vi "BRig_RT__Case_Exp__State_initTrial__LC_ENL__v18.vi"(6 "input_arrTrig":bool[](array[boolean]), 8 "input_dataTrial":u16[][](array[numeric]), 9 "input_dataExp":u16[](array[numeric]), 10 "input_dataLC":u16[](array[numeric]), 11 "input_dataCurrent":u16[](array[numeric])) -> (0 "output_dataTrial":u16[][](array[numeric]), 3 "output_dataCurrent":u16[](array[numeric]), 4 "output_arrTrig":bool[](array[boolean]))   [LabVIEW 2014]
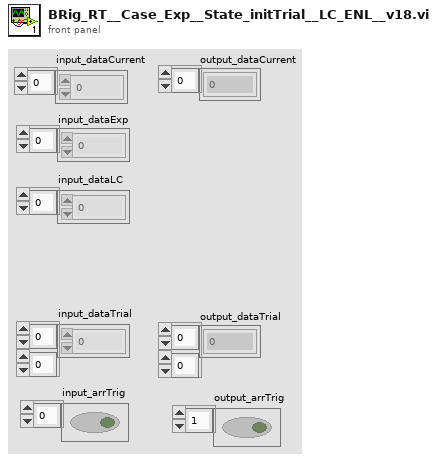
[diagram p1: front panel]
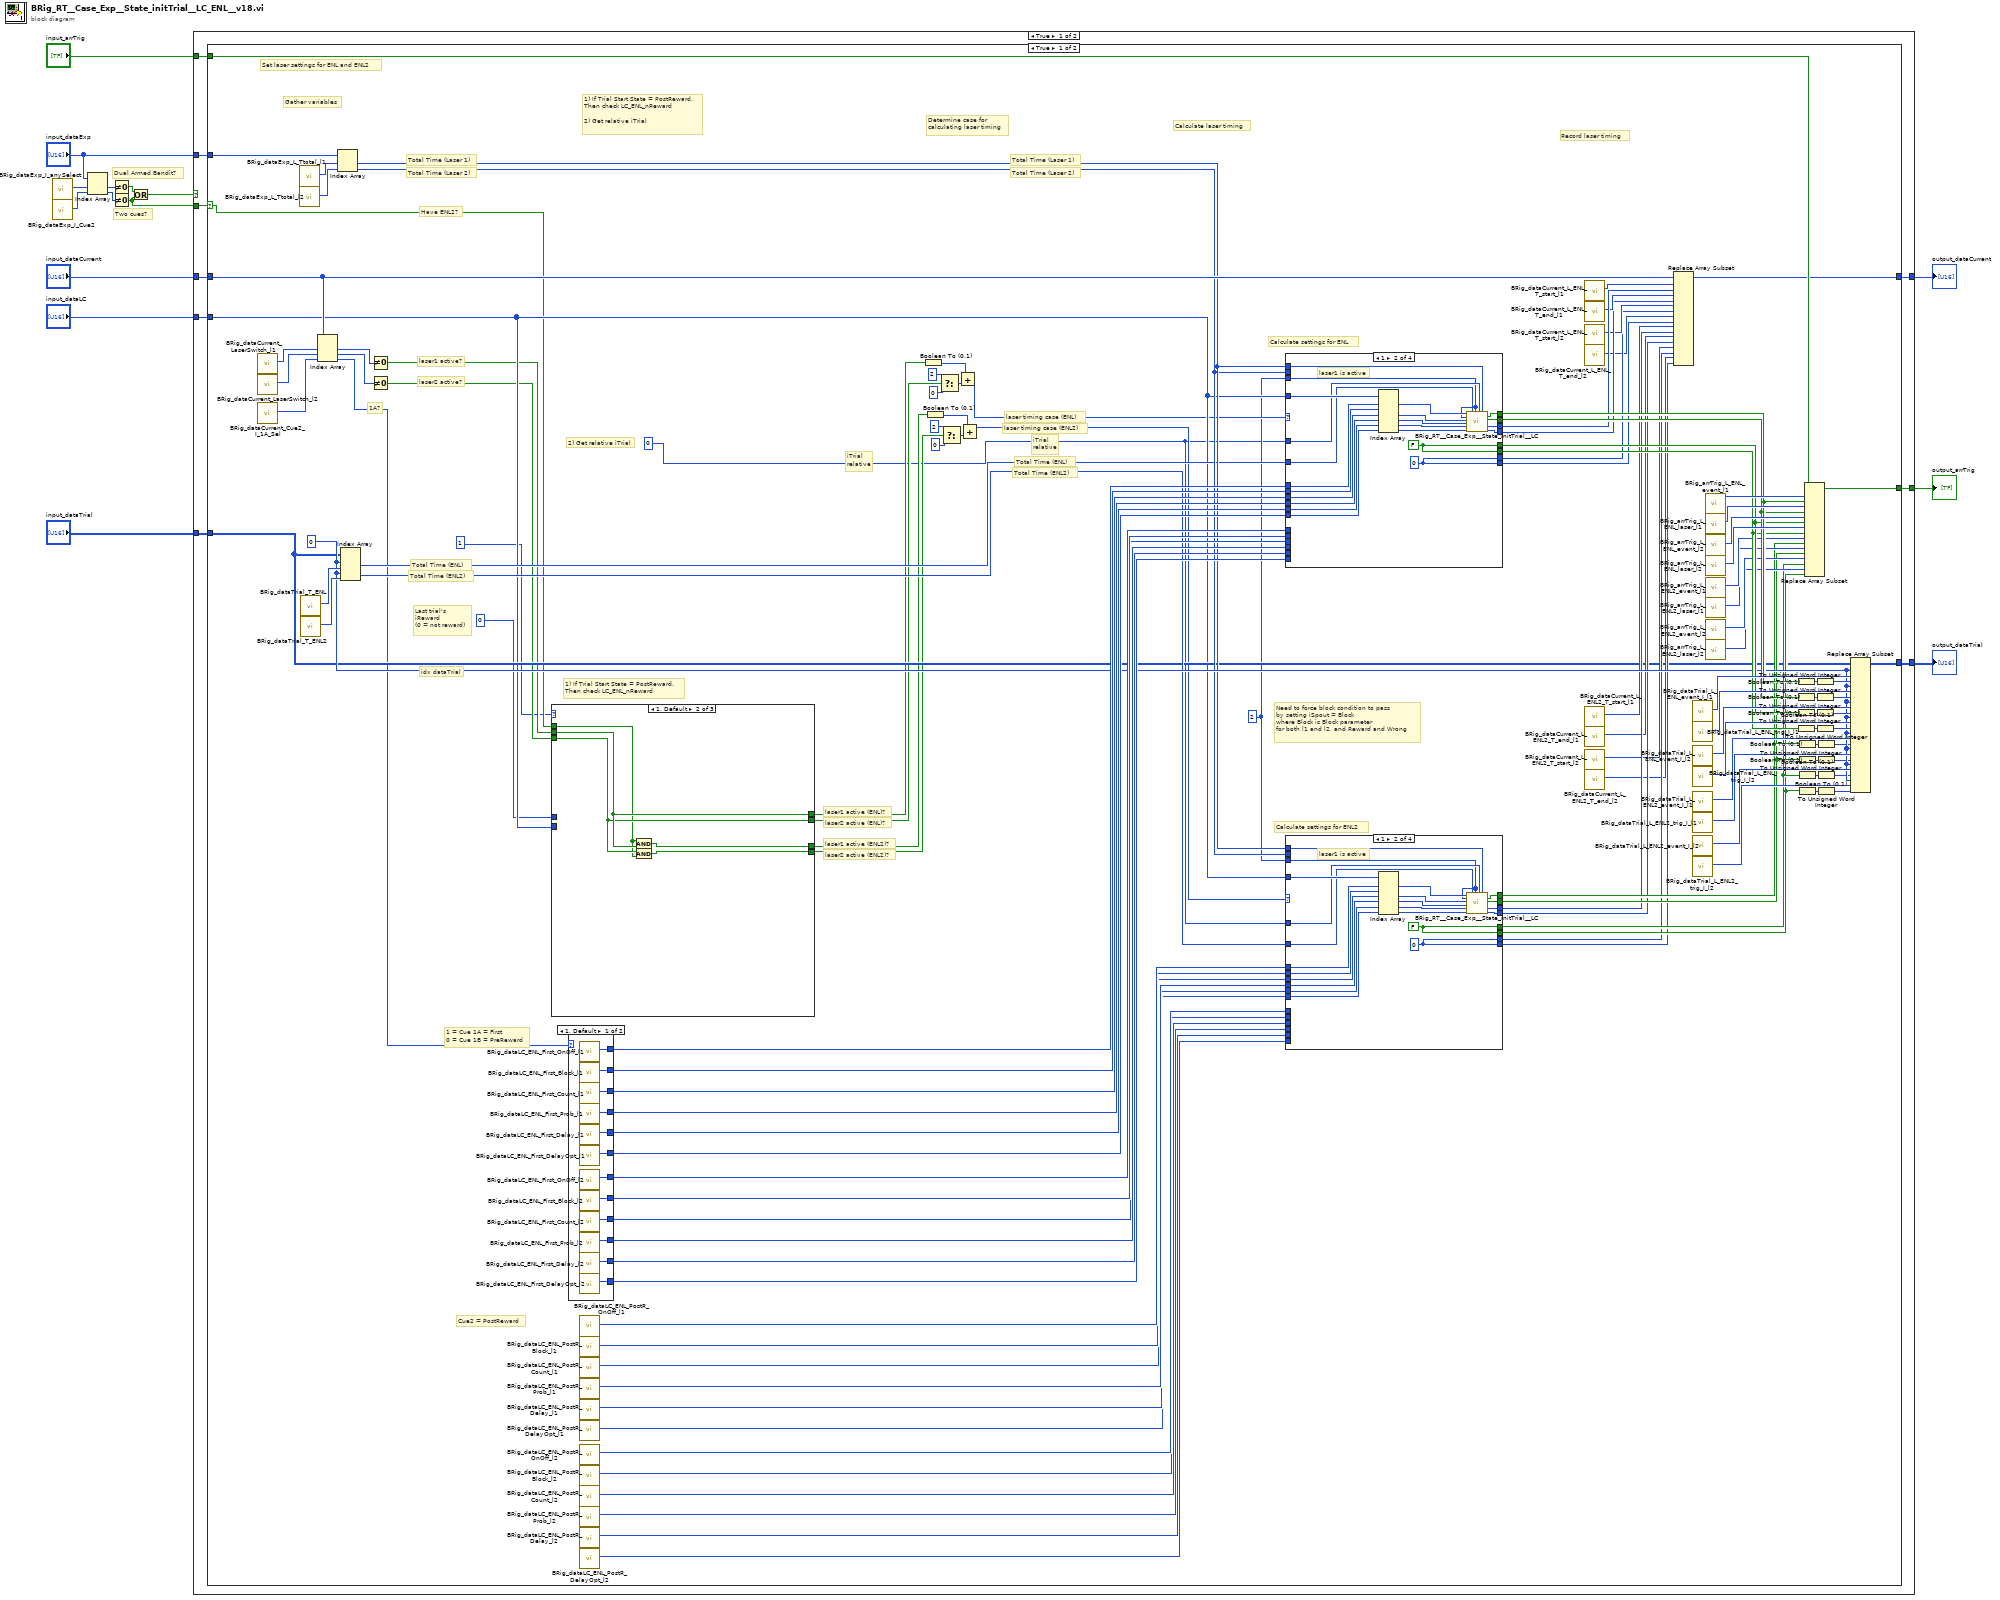
[diagram p0: block diagram]
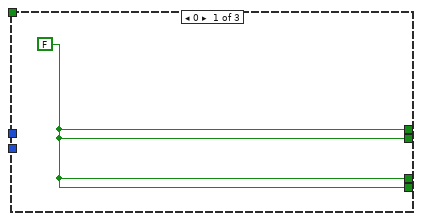
[diagram p2: hidden frame]
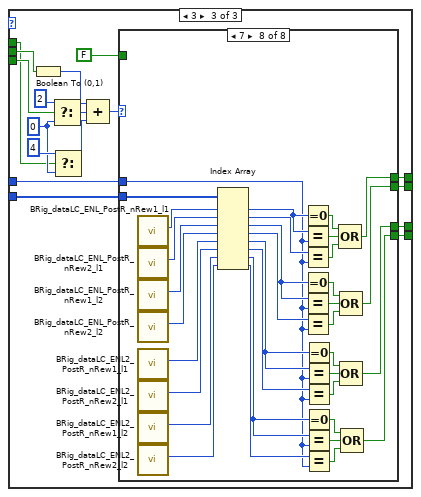
[diagram p3: hidden frame]
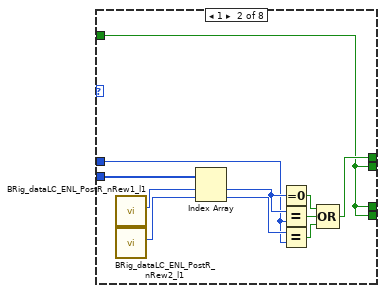
[diagram p5: hidden frame]
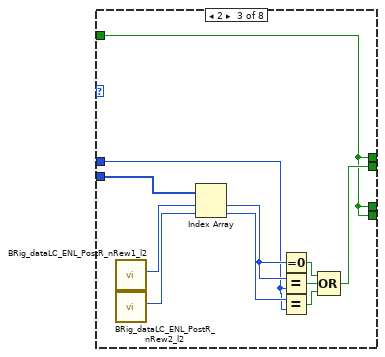
[diagram p6: hidden frame]
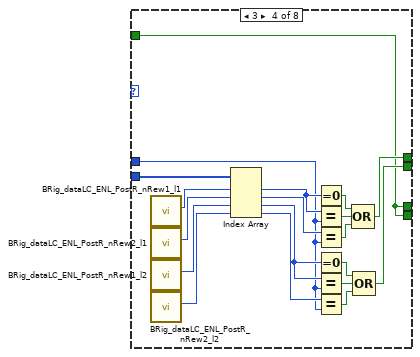
[diagram p7: hidden frame]
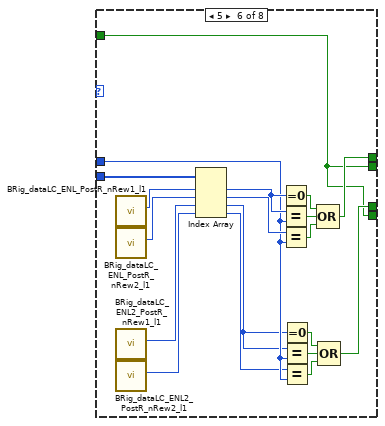
[diagram p9: hidden frame]
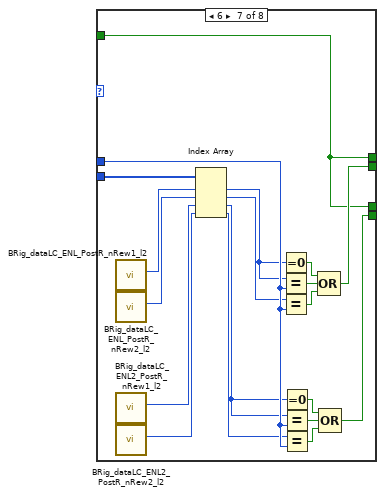
[diagram p10: hidden frame]
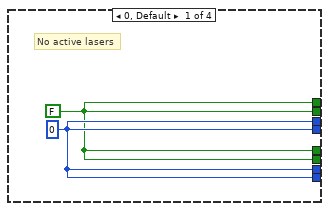
[diagram p11: hidden frame]
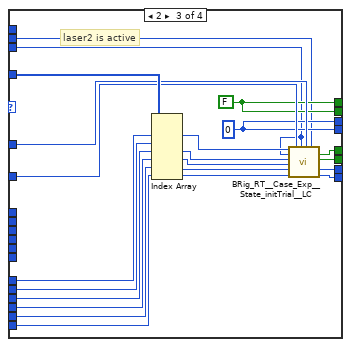
[diagram p12: hidden frame]
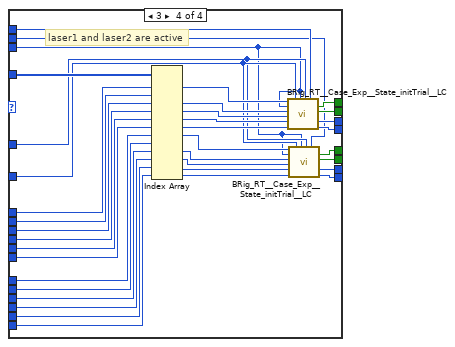
[diagram p13: hidden frame]
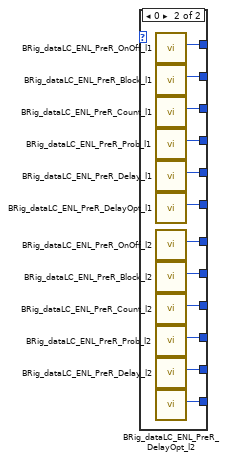
[diagram p14: hidden frame]
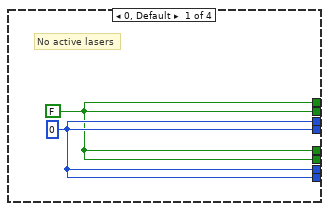
[diagram p15: hidden frame]
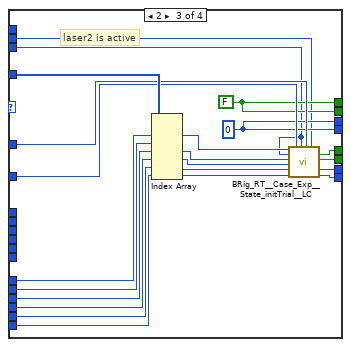
[diagram p16: hidden frame]
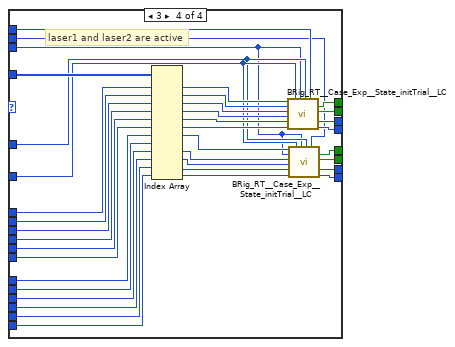
[diagram p17: hidden frame]
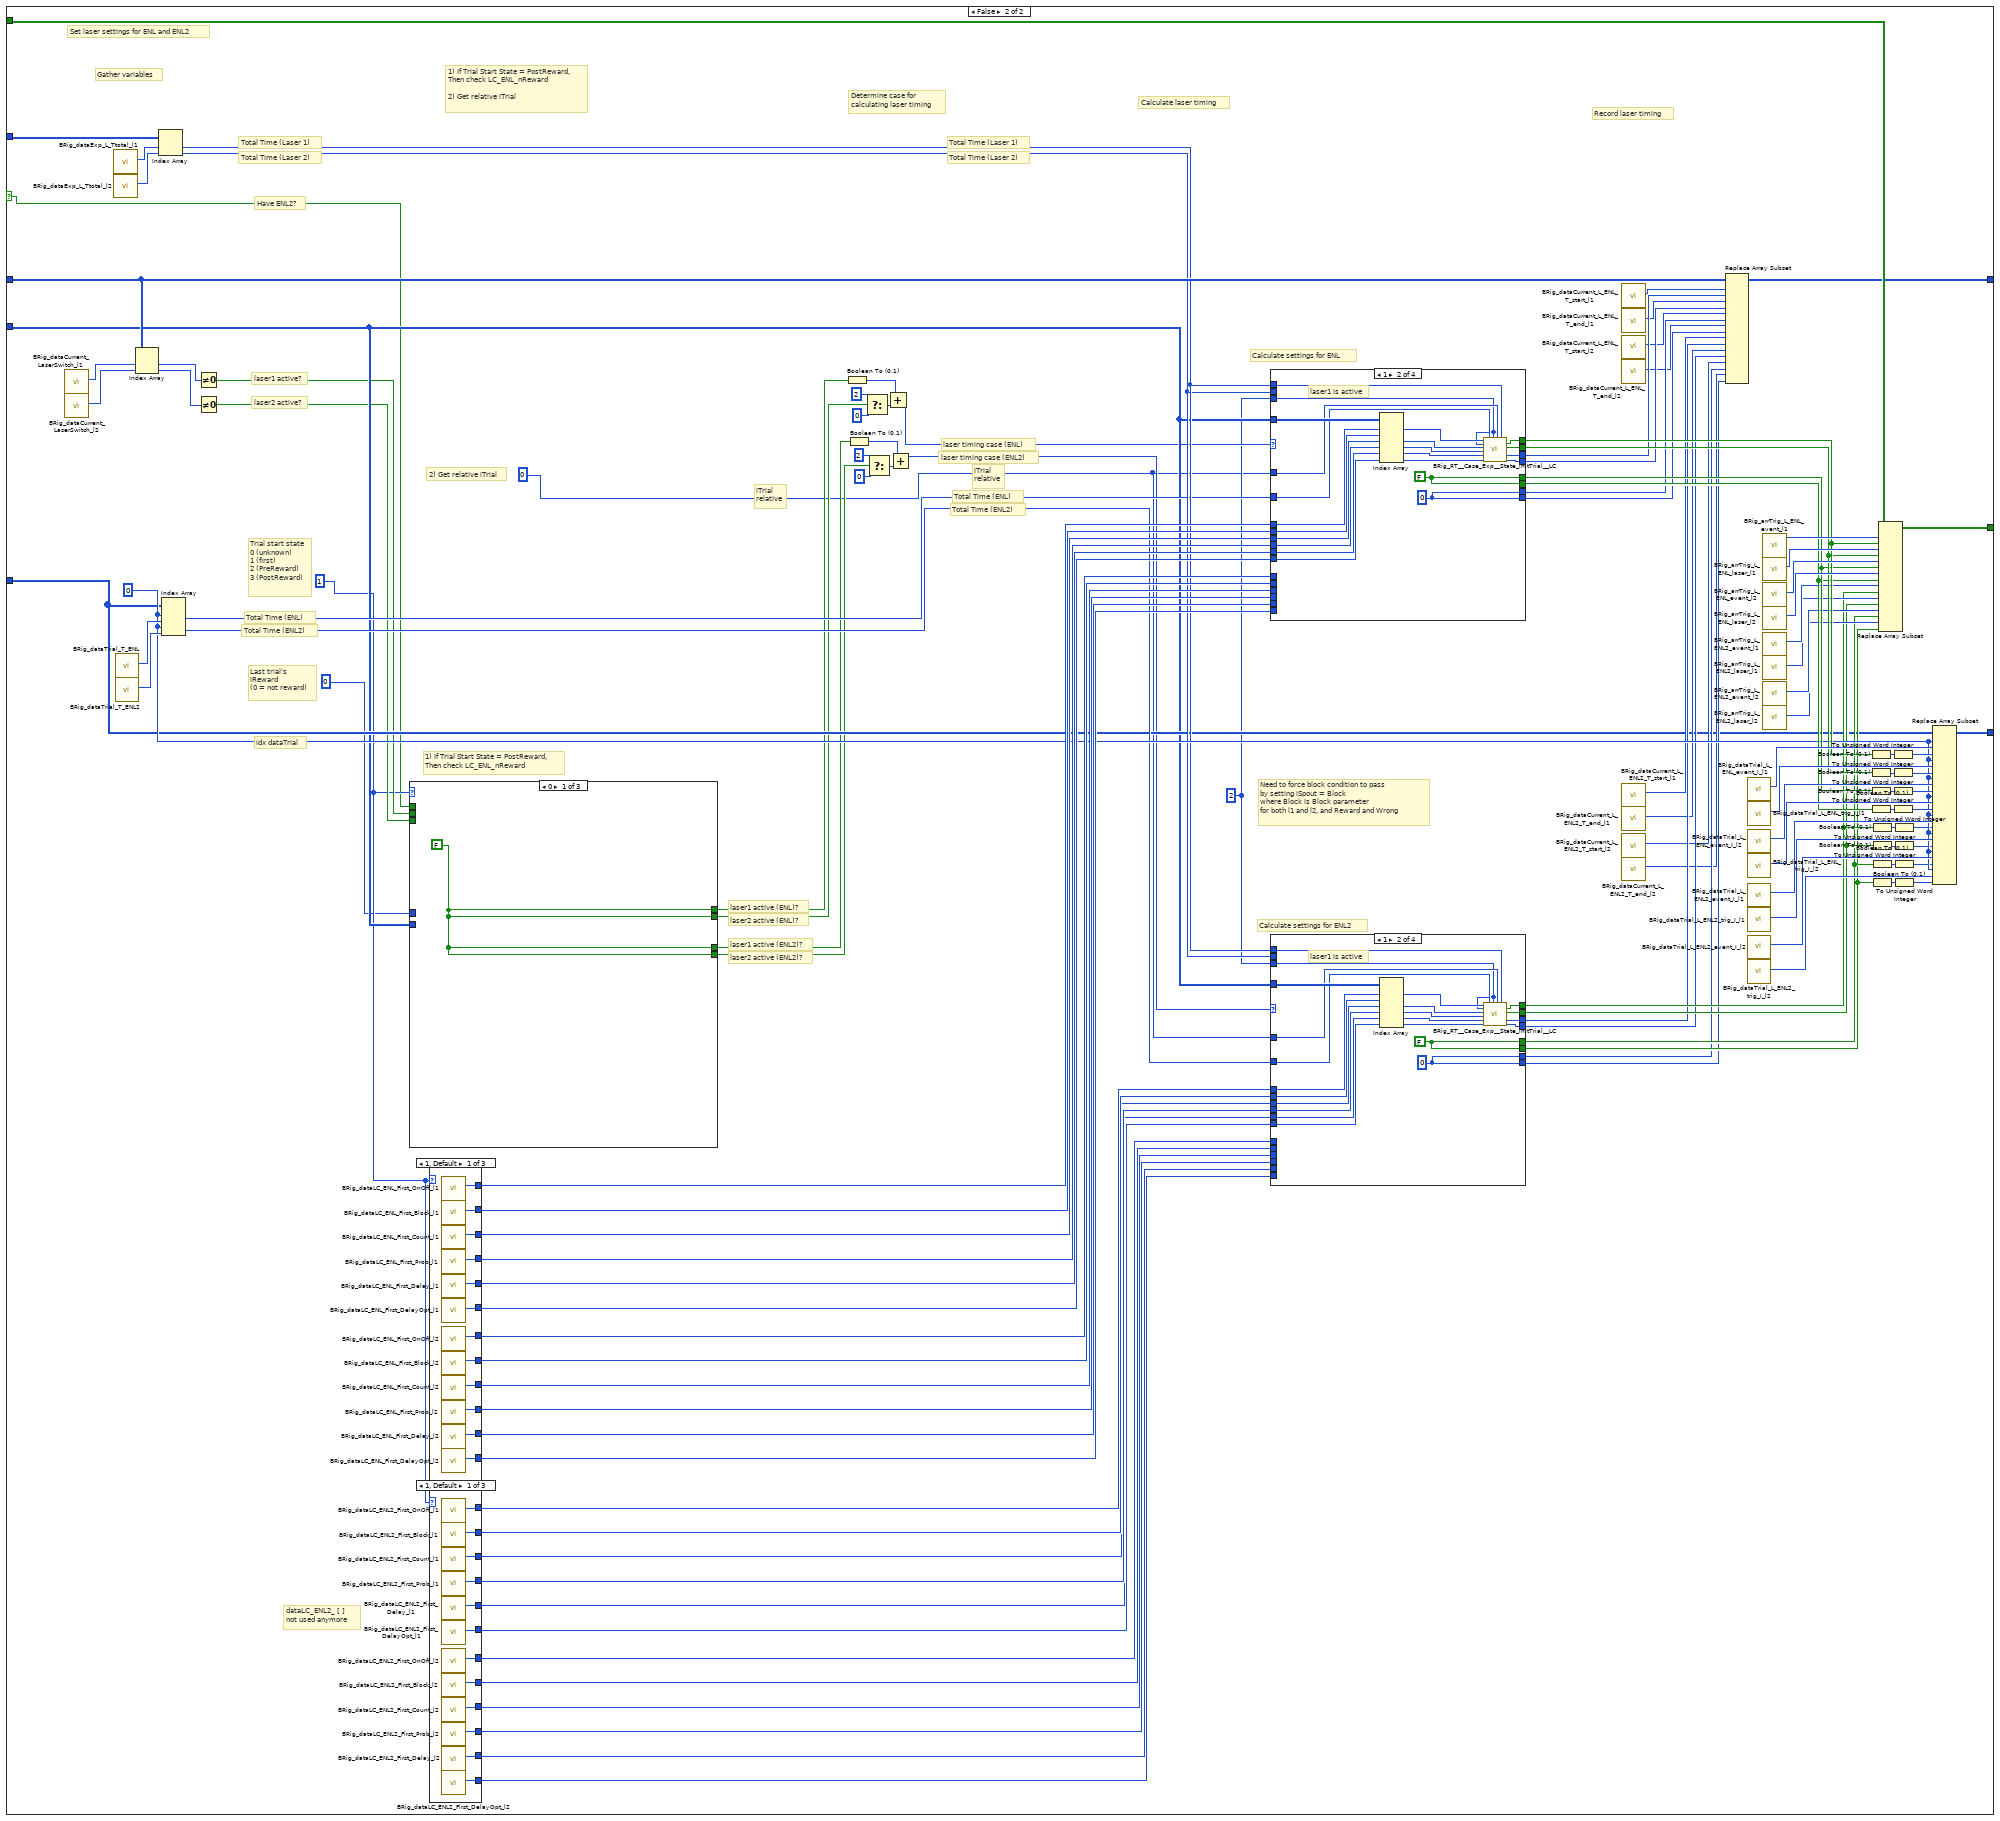
[diagram p18: hidden frame]
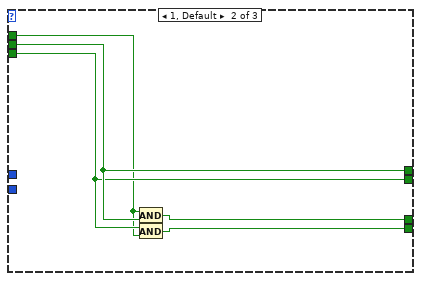
[diagram p19: hidden frame]
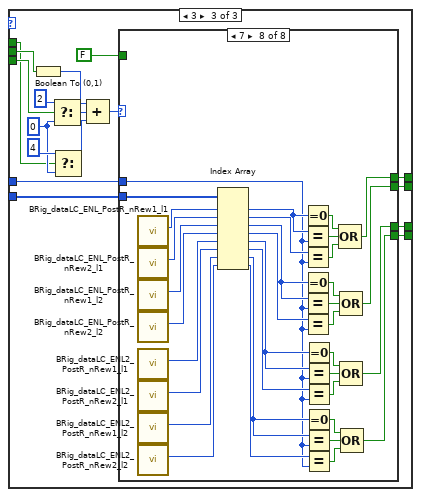
[diagram p20: hidden frame]
diagram:
  # "Two cues?"
  # "Dual Armed Bandit?"
  n1 = call "BRig_dataExp_I_anySelect.vi"() -> ("output_I_anySelect"=w8:i32)  [unwired: 11 in]
  n2 = call "BRig_dataExp_I_Cue2.vi"() -> ("output_I_Cue2"=w6:i32)  [unwired: 11 in]
  n3 = Index Array(array="input_dataExp", index #1=w8, index #2=w6) -> (element #1=w7:u16, element #2=w5:u16)
  n4 = Not Equal To 0?(x=w7) -> (x != 0?=w4:bool)
  n5 = Not Equal To 0?(x=w5) -> (x != 0?=w1:bool)
  n6 = Or(x=w4, y=w1) -> (x .or. y?=w2:bool)
  n7 = case shown="True" w2 {
    tunnel: "input_arrTrig" -> [w24 w1044]
    tunnel: [w23 w1043] -> w14
    tunnel: [w22 w1022] -> w13
    tunnel: "input_dataCurrent" -> [w21 w1021]
    tunnel: [w20 w1020] -> w11
    tunnel: "input_dataExp" -> [w19 w997]
    tunnel: "input_dataTrial" -> [w18 w986]
    tunnel: "input_dataLC" -> [w17 w984]
    tunnel: w1 -> [w16 _]
    frame True {
      n8 = case shown="True" w16 {
        selector: w16 -> [w41 w477]
        tunnel: w24 -> [w140 w589]
        tunnel: [w139 w588] -> w23
        tunnel: [w118 w567] -> w22
        tunnel: w21 -> [w117 w566]
        tunnel: [w116 w565] -> w20
        tunnel: w19 -> [w93 w542]
        tunnel: w18 -> [w57 w494]
        tunnel: w17 -> [w56 w493]
        frame True {
          w42 = u16 0
          w43 = u16 2 ("input_sState_start")
          w79 = 0
          # "Cue2 = PostReward"
          # "1 = Cue 1A = First\n0 = Cue 1B = PreReward"
          # "1A?"
          # "Need to force block condition to pass\nby setting iSpout = Block\nwhere Block is Block parameter\nfor both l1 and l2, and Reward and Wrong"
          # "Record laser timing"
          # "Calculate laser timing"
          # "Total Time (ENL2)"
          # "Total Time (ENL)"
          # "iTrial\nrelative"
          # "Total Time (Laser 2)"
          # "Total Time (Laser 1)"
          # "laser timing case (ENL2)"
          # "Determine case for\ncalculating laser timing"
          # "2) Get relative iTrial"
          # "1) If Trial Start State = PostReward,\nThen check LC_ENL_nReward"
          # "laser2 active (ENL2)?"
          # "laser1 active (ENL2)?"
          # "laser2 active (ENL)?"
          # "laser1 active (ENL)?"
          # "1) If Trial Start State = PostReward,\nThen check LC_ENL_nReward\n\n2) Get relative iTrial"
          # "Gather variables"
          # "Last trial's\niReward\n(0 = not reward)"
          # "idx dataTrial"
          # "Total Time (ENL2)"
          # "Total Time (ENL)"
          # "Have ENL2?"
          # "Total Time (Laser 2)"
          # "Total Time (Laser 1)"
          # "Calculate settings for ENL2"
          # "Calculate settings for ENL"
          # "Set laser settings for ENL and ENL2"
          # "iTrial\nrelative"
          # "laser timing case (ENL)"
          # "laser2 active?"
          # "laser1 active?"
          n9 = call "BRig_dataCurrent_LaserSwitch_l1.vi"() -> ("output_LaserSwitch_l1"=w148:i32)  [unwired: 11 in]
          n10 = call "BRig_dataCurrent_LaserSwitch_l2.vi"() -> ("output_LaserSwitch_l2"=w147:i32)  [unwired: 11 in]
          n11 = call "BRig_dataCurrent_Cue2_I_1A_Sel.vi"() -> ("output_Cue2_I_1A_Sel"=w39:i32)  [unwired: 11 in]
          n12 = call "BRig_dataExp_L_Ttotal_l1.vi"() -> ("output_L_Ttotal_l1"=w94:i32)  [unwired: 11 in]
          n13 = call "BRig_dataExp_L_Ttotal_l2.vi"() -> ("output_L_Ttotal_l2"=w95:i32)  [unwired: 11 in]
          n14 = call "BRig_dataTrial_T_ENL.vi"() -> ("output_T_ENL"=w92:i32)  [unwired: 11 in]
          n15 = call "BRig_dataTrial_T_ENL2.vi"() -> ("output_T_ENL2"=w91:i32)  [unwired: 11 in]
          n16 = Index Array(array=w117, index #1=w148, index #2=w147, index #3=w39) -> (element #1=w146:u16, element #2=w145:u16, element #3=w38:u16)
          n17 = Index Array(array=w93, index #1=w94, index #2=w95) -> (element #1=w73:u16, element #2=w72:u16)
          n18 = Index Array(array=w57, index (row) #1=w79, index (col) #1=w92, index (row) #2=w79, index (col) #2=w91) -> (element #1=w59:u16, element #2=w58:u16)
          n19 = Not Equal To 0?(x=w146) -> (x != 0?=w54:bool)
          n20 = Not Equal To 0?(x=w145) -> (x != 0?=w55:bool)
          n21 = case shown="1, Default" u16 1 {
            tunnel: u16 0 -> [_ _ w163]
            tunnel: w56 -> [_ _ w164]
            tunnel: w55 -> [_ w153 w156]
            tunnel: w54 -> [_ w154 w157]
            tunnel: w41 -> [_ w152 w155]
            tunnel: [w149 w154 w162] -> w53
            tunnel: [w149 w153 w161] -> w52
            tunnel: [w149 w151 w160] -> w47
            tunnel: [w149 w150 w159] -> w46
            frame 0 {
              w149 = FALSE
            }
            frame 1, Default {
              n22 = And(x=w152, y=w154) -> (x .and. y?=w151:bool)
              n23 = And(x=w153, y=w152) -> (x .and. y?=w150:bool)
            }
            frame 3 {
              w169 = i16 0 ("f")
              n24 = Boolean To (0,1)(Boolean=w157) -> (0, 1=w167:i16)
              n25 = Select(t=i16 2, s=w156, f=w169) -> (s? t:f=w168:i16)
              n26 = Select(t=i16 4, s=w155, f=w169) -> (s? t:f=w166:i16)
              n27 = Compound Arithmetic op=ADD(w167, w168, w166) -> (w165:i16)
              n28 = case shown="7" w165 {
                tunnel: w164 -> [_ w176 w187 w199 _ w226 w249 w272]
                tunnel: w163 -> [_ w175 w186 w198 _ w222 w245 w257]
                tunnel: [w172 w174 w184 w197 w214 w221 w242 w256] -> w162
                tunnel: [w172 w173 w185 w196 w214 w219 w244 w255] -> w161
                tunnel: [w172 w173 w184 w195 w214 w220 w242 w254] -> w160
                tunnel: [w172 w173 w184 w195 w214 w219 w243 w253] -> w159
                tunnel: FALSE -> [w172 w173 w184 w195 w214 w219 w242 _]
                frame 0, Default {
                }
                frame 1 {
                  n29 = call "BRig_dataLC_ENL_PostR_nRew1_l1.vi"() -> ("output_ENL_PostR_nRew1_l1"=w183:i32)  [unwired: 11 in]
                  n30 = call "BRig_dataLC_ENL_PostR_nRew2_l1.vi"() -> ("output_ENL_PostR_nRew2_l1"=w182:i32)  [unwired: 11 in]
                  n31 = Index Array(array=w176, index #1=w183, index #2=w182) -> (element #1=w178:u16, element #2=w177:u16)
                  n32 = Equal To 0?(x=w178) -> (x = 0?=w179:bool)
                  n33 = Equal?(x=w178, y=w175) -> (x = y?=w180:bool)
                  n34 = Equal?(x=w177, y=w175) -> (x = y?=w181:bool)
                  n35 = Compound Arithmetic op=OR(w179, w180, w181) -> (w174:bool)
                }
                frame 2 {
                  n36 = call "BRig_dataLC_ENL_PostR_nRew1_l2.vi"() -> ("output_ENL_PostR_nRew1_l2"=w194:i32)  [unwired: 11 in]
                  n37 = call "BRig_dataLC_ENL_PostR_nRew2_l2.vi"() -> ("output_ENL_PostR_nRew2_l2"=w193:i32)  [unwired: 11 in]
                  n38 = Index Array(array=w187, index #1=w194, index #2=w193) -> (element #1=w188:u16, element #2=w189:u16)
                  n39 = Equal To 0?(x=w188) -> (x = 0?=w191:bool)
                  n40 = Equal?(x=w188, y=w186) -> (x = y?=w190:bool)
                  n41 = Equal?(x=w189, y=w186) -> (x = y?=w192:bool)
                  n42 = Compound Arithmetic op=OR(w191, w190, w192) -> (w185:bool)
                }
                frame 3 {
                  n43 = call "BRig_dataLC_ENL_PostR_nRew1_l1.vi"() -> ("output_ENL_PostR_nRew1_l1"=w213:i32)  [unwired: 11 in]
                  n44 = call "BRig_dataLC_ENL_PostR_nRew2_l1.vi"() -> ("output_ENL_PostR_nRew2_l1"=w212:i32)  [unwired: 11 in]
                  n45 = call "BRig_dataLC_ENL_PostR_nRew1_l2.vi"() -> ("output_ENL_PostR_nRew1_l2"=w211:i32)  [unwired: 11 in]
                  n46 = call "BRig_dataLC_ENL_PostR_nRew2_l2.vi"() -> ("output_ENL_PostR_nRew2_l2"=w210:i32)  [unwired: 11 in]
                  n47 = Index Array(array=w199, index #1=w213, index #2=w212, index #3=w211, index #4=w210) -> (element #1=w203:u16, element #2=w202:u16, element #3=w200:u16, element #4=w201:u16)
                  n48 = Equal To 0?(x=w203) -> (x = 0?=w204:bool)
                  n49 = Equal?(x=w203, y=w198) -> (x = y?=w205:bool)
                  n50 = Equal?(x=w202, y=w198) -> (x = y?=w206:bool)
                  n51 = Equal To 0?(x=w200) -> (x = 0?=w208:bool)
                  n52 = Equal?(x=w200, y=w198) -> (x = y?=w207:bool)
                  n53 = Equal?(x=w201, y=w198) -> (x = y?=w209:bool)
                  n54 = Compound Arithmetic op=OR(w204, w205, w206) -> (w197:bool)
                  n55 = Compound Arithmetic op=OR(w208, w207, w209) -> (w196:bool)
                }
                frame 4 {
                }
                frame 5 {
                  n56 = call "BRig_dataLC_ENL_PostR_nRew1_l1.vi"() -> ("output_ENL_PostR_nRew1_l1"=w233:i32)  [unwired: 11 in]
                  n57 = call "BRig_dataLC_ENL_PostR_nRew2_l1.vi"() -> ("output_ENL_PostR_nRew2_l1"=w232:i32)  [unwired: 11 in]
                  n58 = call "BRig_dataLC_ENL2_PostR_nRew1_l1.vi"() -> ("output_ENL2_PostR_nRew1_l1"=w218:i32)  [unwired: 11 in]
                  n59 = call "BRig_dataLC_ENL2_PostR_nRew2_l1.vi"() -> ("output_ENL2_PostR_nRew2_l1"=w217:i32)  [unwired: 11 in]
                  n60 = Index Array(array=w226, index #1=w233, index #2=w232, index #3=w218, index #4=w217) -> (element #1=w228:u16, element #2=w227:u16, element #3=w216:u16, element #4=w215:u16)
                  n61 = Equal To 0?(x=w228) -> (x = 0?=w229:bool)
                  n62 = Equal?(x=w228, y=w222) -> (x = y?=w230:bool)
                  n63 = Equal?(x=w227, y=w222) -> (x = y?=w231:bool)
                  n64 = Equal To 0?(x=w216) -> (x = 0?=w225:bool)
                  n65 = Equal?(x=w216, y=w222) -> (x = y?=w224:bool)
                  n66 = Equal?(x=w215, y=w222) -> (x = y?=w223:bool)
                  n67 = Compound Arithmetic op=OR(w229, w230, w231) -> (w221:bool)
                  n68 = Compound Arithmetic op=OR(w225, w224, w223) -> (w220:bool)
                }
                frame 6 {
                  n69 = call "BRig_dataLC_ENL_PostR_nRew1_l2.vi"() -> ("output_ENL_PostR_nRew1_l2"=w241:i32)  [unwired: 11 in]
                  n70 = call "BRig_dataLC_ENL_PostR_nRew2_l2.vi"() -> ("output_ENL_PostR_nRew2_l2"=w240:i32)  [unwired: 11 in]
                  n71 = call "BRig_dataLC_ENL2_PostR_nRew1_l2.vi"() -> ("output_ENL2_PostR_nRew1_l2"=w237:i32)  [unwired: 11 in]
                  n72 = call "BRig_dataLC_ENL2_PostR_nRew2_l2.vi"() -> ("output_ENL2_PostR_nRew2_l2"=w236:i32)  [unwired: 11 in]
                  n73 = Index Array(array=w249, index #1=w241, index #2=w240, index #3=w237, index #4=w236) -> (element #1=w239:u16, element #2=w238:u16, element #3=w235:u16, element #4=w234:u16)
                  n74 = Equal To 0?(x=w239) -> (x = 0?=w251:bool)
                  n75 = Equal?(x=w239, y=w245) -> (x = y?=w250:bool)
                  n76 = Equal?(x=w238, y=w245) -> (x = y?=w252:bool)
                  n77 = Equal To 0?(x=w235) -> (x = 0?=w247:bool)
                  n78 = Equal?(x=w235, y=w245) -> (x = y?=w248:bool)
                  n79 = Equal?(x=w234, y=w245) -> (x = y?=w246:bool)
                  n80 = Compound Arithmetic op=OR(w251, w250, w252) -> (w244:bool)
                  n81 = Compound Arithmetic op=OR(w247, w248, w246) -> (w243:bool)
                }
                frame 7 {
                  n82 = call "BRig_dataLC_ENL_PostR_nRew1_l1.vi"() -> ("output_ENL_PostR_nRew1_l1"=w286:i32)  [unwired: 11 in]
                  n83 = call "BRig_dataLC_ENL_PostR_nRew2_l1.vi"() -> ("output_ENL_PostR_nRew2_l1"=w285:i32)  [unwired: 11 in]
                  n84 = call "BRig_dataLC_ENL_PostR_nRew1_l2.vi"() -> ("output_ENL_PostR_nRew1_l2"=w284:i32)  [unwired: 11 in]
                  n85 = call "BRig_dataLC_ENL_PostR_nRew2_l2.vi"() -> ("output_ENL_PostR_nRew2_l2"=w283:i32)  [unwired: 11 in]
                  n86 = call "BRig_dataLC_ENL2_PostR_nRew1_l1.vi"() -> ("output_ENL2_PostR_nRew1_l1"=w271:i32)  [unwired: 11 in]
                  n87 = call "BRig_dataLC_ENL2_PostR_nRew2_l1.vi"() -> ("output_ENL2_PostR_nRew2_l1"=w270:i32)  [unwired: 11 in]
                  n88 = call "BRig_dataLC_ENL2_PostR_nRew1_l2.vi"() -> ("output_ENL2_PostR_nRew1_l2"=w269:i32)  [unwired: 11 in]
                  n89 = call "BRig_dataLC_ENL2_PostR_nRew2_l2.vi"() -> ("output_ENL2_PostR_nRew2_l2"=w268:i32)  [unwired: 11 in]
                  n90 = Index Array(array=w272, index #1=w286, index #2=w285, index #3=w284, index #4=w283, index #5=w271, index #6=w270, index #7=w269, index #8=w268) -> (element #1=w276:u16, element #2=w275:u16, element #3=w273:u16, element #4=w274:u16, element #5=w261:u16, element #6=w260:u16, element #7=w258:u16, element #8=w259:u16)
                  n91 = Equal To 0?(x=w276) -> (x = 0?=w277:bool)
                  n92 = Equal?(x=w276, y=w257) -> (x = y?=w278:bool)
                  n93 = Equal?(x=w275, y=w257) -> (x = y?=w279:bool)
                  n94 = Equal To 0?(x=w273) -> (x = 0?=w281:bool)
                  n95 = Equal?(x=w273, y=w257) -> (x = y?=w280:bool)
                  n96 = Equal?(x=w274, y=w257) -> (x = y?=w282:bool)
                  n97 = Equal To 0?(x=w261) -> (x = 0?=w267:bool)
                  n98 = Equal?(x=w261, y=w257) -> (x = y?=w266:bool)
                  n99 = Equal?(x=w260, y=w257) -> (x = y?=w265:bool)
                  n100 = Equal To 0?(x=w258) -> (x = 0?=w263:bool)
                  n101 = Equal?(x=w258, y=w257) -> (x = y?=w264:bool)
                  n102 = Equal?(x=w259, y=w257) -> (x = y?=w262:bool)
                  n103 = Compound Arithmetic op=OR(w277, w278, w279) -> (w256:bool)
                  n104 = Compound Arithmetic op=OR(w281, w280, w282) -> (w255:bool)
                  n105 = Compound Arithmetic op=OR(w267, w266, w265) -> (w254:bool)
                  n106 = Compound Arithmetic op=OR(w263, w264, w262) -> (w253:bool)
                }
              }
            }
          }
          n107 = case shown="1, Default" w38 {
            tunnel: [w380 w392] -> w107
            tunnel: [w379 w391] -> w106
            tunnel: [w378 w390] -> w105
            tunnel: [w377 w389] -> w104
            tunnel: [w376 w388] -> w103
            tunnel: [w375 w387] -> w102
            tunnel: [w374 w386] -> w101
            tunnel: [w373 w385] -> w100
            tunnel: [w372 w384] -> w99
            tunnel: [w371 w383] -> w98
            tunnel: [w370 w382] -> w97
            tunnel: [w369 w381] -> w96
            frame 1, Default {
              n108 = call "BRig_dataLC_ENL_First_OnOff_l1.vi"() -> ("output_ENL_First_OnOff"=w380:i32)  [unwired: 11 in]
              n109 = call "BRig_dataLC_ENL_First_Block_l1.vi"() -> ("output_ENL_First_Block"=w379:i32)  [unwired: 11 in]
              n110 = call "BRig_dataLC_ENL_First_Count_l1.vi"() -> ("output_ENL_First_Count"=w378:i32)  [unwired: 11 in]
              n111 = call "BRig_dataLC_ENL_First_Prob_l1.vi"() -> ("output_ENL_First_Prob"=w377:i32)  [unwired: 11 in]
              n112 = call "BRig_dataLC_ENL_First_Delay_l1.vi"() -> ("output_ENL_First_Delay"=w376:i32)  [unwired: 11 in]
              n113 = call "BRig_dataLC_ENL_First_DelayOpt_l1.vi"() -> ("output_ENL_First_DelayOpt"=w375:i32)  [unwired: 11 in]
              n114 = call "BRig_dataLC_ENL_First_OnOff_l2.vi"() -> ("output_ENL_First_OnOff_l2"=w374:i32)  [unwired: 11 in]
              n115 = call "BRig_dataLC_ENL_First_Block_l2.vi"() -> ("output_ENL_First_Block_l2"=w373:i32)  [unwired: 11 in]
              n116 = call "BRig_dataLC_ENL_First_Count_l2.vi"() -> ("output_ENL_First_Count_l2"=w372:i32)  [unwired: 11 in]
              n117 = call "BRig_dataLC_ENL_First_Prob_l2.vi"() -> ("output_ENL_First_Prob_l2"=w371:i32)  [unwired: 11 in]
              n118 = call "BRig_dataLC_ENL_First_Delay_l2.vi"() -> ("output_ENL_First_Delay_l2"=w370:i32)  [unwired: 11 in]
              n119 = call "BRig_dataLC_ENL_First_DelayOpt_l2.vi"() -> ("output_ENL_First_DelayOpt_l2"=w369:i32)  [unwired: 11 in]
            }
            frame 0 {
              n120 = call "BRig_dataLC_ENL_PreR_OnOff_l1.vi"() -> ("output_ENL_PreR_OnOff"=w392:i32)  [unwired: 11 in]
              n121 = call "BRig_dataLC_ENL_PreR_Block_l1.vi"() -> ("output_ENL_PreR_Block"=w391:i32)  [unwired: 11 in]
              n122 = call "BRig_dataLC_ENL_PreR_Count_l1.vi"() -> ("output_ENL_PreR_Count"=w390:i32)  [unwired: 11 in]
              n123 = call "BRig_dataLC_ENL_PreR_Prob_l1.vi"() -> ("output_ENL_PreR_Prob"=w389:i32)  [unwired: 11 in]
              n124 = call "BRig_dataLC_ENL_PreR_Delay_l1.vi"() -> ("output_ENL_PreR_Delay"=w388:i32)  [unwired: 11 in]
              n125 = call "BRig_dataLC_ENL_PreR_DelayOpt_l1.vi"() -> ("output_ENL_PreR_DelayOpt"=w387:i32)  [unwired: 11 in]
              n126 = call "BRig_dataLC_ENL_PreR_OnOff_l2.vi"() -> ("output_ENL_PreR_OnOff_l2"=w386:i32)  [unwired: 11 in]
              n127 = call "BRig_dataLC_ENL_PreR_Block_l2.vi"() -> ("output_ENL_PreR_Block_l2"=w385:i32)  [unwired: 11 in]
              n128 = call "BRig_dataLC_ENL_PreR_Count_l2.vi"() -> ("output_ENL_PreR_Count_l2"=w384:i32)  [unwired: 11 in]
              n129 = call "BRig_dataLC_ENL_PreR_Prob_l2.vi"() -> ("output_ENL_PreR_Prob_l2"=w383:i32)  [unwired: 11 in]
              n130 = call "BRig_dataLC_ENL_PreR_Delay_l2.vi"() -> ("output_ENL_PreR_Delay_l2"=w382:i32)  [unwired: 11 in]
              n131 = call "BRig_dataLC_ENL_PreR_DelayOpt_l2.vi"() -> ("output_ENL_PreR_DelayOpt_l2"=w381:i32)  [unwired: 11 in]
            }
          }
          n132 = call "BRig_dataLC_ENL_PostR_OnOff_l1.vi"() -> ("output_ENL_PostR_OnOff"=w36:i32)  [unwired: 11 in]
          n133 = call "BRig_dataLC_ENL_PostR_Block_l1.vi"() -> ("output_ENL_PostR_Block"=w35:i32)  [unwired: 11 in]
          n134 = call "BRig_dataLC_ENL_PostR_Count_l1.vi"() -> ("output_ENL_PostR_Count"=w34:i32)  [unwired: 11 in]
          n135 = call "BRig_dataLC_ENL_PostR_Prob_l1.vi"() -> ("output_ENL_PostR_Prob"=w33:i32)  [unwired: 11 in]
          n136 = call "BRig_dataLC_ENL_PostR_Delay_l1.vi"() -> ("output_ENL_PostR_Delay"=w32:i32)  [unwired: 11 in]
          n137 = call "BRig_dataLC_ENL_PostR_DelayOpt_l1.vi"() -> ("output_ENL_PostR_DelayOpt"=w31:i32)  [unwired: 11 in]
          n138 = call "BRig_dataLC_ENL_PostR_OnOff_l2.vi"() -> ("output_ENL_PostR_OnOff_l2"=w30:i32)  [unwired: 11 in]
          n139 = call "BRig_dataLC_ENL_PostR_Block_l2.vi"() -> ("output_ENL_PostR_Block_l2"=w29:i32)  [unwired: 11 in]
          n140 = call "BRig_dataLC_ENL_PostR_Count_l2.vi"() -> ("output_ENL_PostR_Count_l2"=w28:i32)  [unwired: 11 in]
          n141 = call "BRig_dataLC_ENL_PostR_Prob_l2.vi"() -> ("output_ENL_PostR_Prob_l2"=w27:i32)  [unwired: 11 in]
          n142 = call "BRig_dataLC_ENL_PostR_Delay_l2.vi"() -> ("output_ENL_PostR_Delay_l2"=w26:i32)  [unwired: 11 in]
          n143 = call "BRig_dataLC_ENL_PostR_DelayOpt_l2.vi"() -> ("output_ENL_PostR_DelayOpt_l2"=w25:i32)  [unwired: 11 in]
          n144 = Boolean To (0,1)(Boolean=w53) -> (0, 1=w142:i16)
          n145 = Boolean To (0,1)(Boolean=w47) -> (0, 1=w50:i16)
          n146 = Select(t=i16 2, s=w52, f=i16 0) -> (s? t:f=w143:i16)
          n147 = Select(t=i16 2, s=w46, f=i16 0) -> (s? t:f=w49:i16)
          n148 = Add(x=w142, y=w143) -> (x+y=w45:i16)
          n149 = Add(x=w50, y=w49) -> (x+y=w44:i16)
          n150 = case shown="1" w45 {
            tunnel: w56 -> [_ w416 w438 w475]
            tunnel: w43 -> [_ w395 w417 w439]
            tunnel: w59 -> [_ w410 w432 w463]
            tunnel: w42 -> [_ w409 w431 w462]
            tunnel: [w393 w408 w420 w461] -> w129
            tunnel: [w393 w407 w420 w460] -> w123
            tunnel: [w394 w406 w419 w459] -> w114
            tunnel: [w394 w405 w419 w458] -> w112
            tunnel: [w393 w398 w430 w457] -> w119
            tunnel: [w394 w397 w429 w456] -> w110
            tunnel: [w393 w398 w428 w455] -> w121
            tunnel: [w394 w397 w427 w454] -> w108
            tunnel: w107 -> [_ w404 _ w453]
            tunnel: w106 -> [_ w403 _ w452]
            tunnel: w105 -> [_ w402 _ w451]
            tunnel: w104 -> [_ w401 _ w450]
            tunnel: w103 -> [_ w400 _ w449]
            tunnel: w102 -> [_ w399 _ w448]
            tunnel: w101 -> [_ _ w426 w447]
            tunnel: w100 -> [_ _ w425 w446]
            tunnel: w99 -> [_ _ w424 w445]
            tunnel: w98 -> [_ _ w423 w444]
            tunnel: w97 -> [_ _ w422 w443]
            tunnel: w96 -> [_ _ w421 w442]
            tunnel: w73 -> [_ w396 _ w441]
            tunnel: w72 -> [_ _ w418 w440]
            frame 0, Default {
              w394 = u16 0
              w393 = FALSE
              # "No active lasers"
            }
            frame 1 {
              w397 = u16 0
              w398 = FALSE
              # "laser1 is active"
              n151 = Index Array(array=w416, index #1=w404, index #2=w403, index #3=w402, index #4=w401, index #5=w400, index #6=w399) -> (element #1=w415:u16, element #3=w414:u16, element #4=w413:u16, element #5=w412:u16, element #6=w411:u16)  [unwired: 1 out]
              n152 = call "BRig_RT__Case_Exp__State_initTrial__LC.vi"("input_L_OnOff"=w415, "input_L_Block"=w395, "input_L_Count"=w414, "input_L_Prob"=w413, "input_L_Tdelay"=w412, "input_L_delayOpt"=w411, "input_T_state"=w410, "input_iSpout"=w395, "input_iTrial_relative"=w409, "input_L_T"=w396) -> ("output_LC_Event"=w408:bool, "output_LC_Laser"=w407:bool, "output_L_Tstart"=w406:u16, "output_L_Tend"=w405:u16)  [unwired: 6 in]
            }
            frame 2 {
              w419 = u16 0
              w420 = FALSE
              # "laser2 is active"
              n153 = Index Array(array=w438, index #1=w426, index #2=w425, index #3=w424, index #4=w423, index #5=w422, index #6=w421) -> (element #1=w433:u16, element #3=w434:u16, element #4=w435:u16, element #5=w436:u16, element #6=w437:u16)  [unwired: 1 out]
              n154 = call "BRig_RT__Case_Exp__State_initTrial__LC.vi"("input_L_OnOff"=w433, "input_L_Block"=w417, "input_L_Count"=w434, "input_L_Prob"=w435, "input_L_Tdelay"=w436, "input_L_delayOpt"=w437, "input_T_state"=w432, "input_iSpout"=w417, "input_iTrial_relative"=w431, "input_L_T"=w418) -> ("output_LC_Event"=w428:bool, "output_LC_Laser"=w430:bool, "output_L_Tstart"=w429:u16, "output_L_Tend"=w427:u16)  [unwired: 6 in]
            }
            frame 3 {
              # "laser1 and laser2 are active"
              n155 = Index Array(array=w475, index #1=w453, index #2=w452, index #3=w451, index #4=w450, index #5=w449, index #6=w448, index #7=w447, index #8=w446, index #9=w445, index #10=w444, index #11=w443, index #12=w442) -> (element #1=w474:u16, element #2=w473:u16, element #3=w472:u16, element #4=w471:u16, element #5=w470:u16, element #6=w469:u16, element #7=w464:u16, element #9=w465:u16, element #10=w466:u16, element #11=w467:u16, element #12=w468:u16)  [unwired: 1 out]
              n156 = call "BRig_RT__Case_Exp__State_initTrial__LC.vi"("input_L_OnOff"=w474, "input_L_Block"=w473, "input_L_Count"=w472, "input_L_Prob"=w471, "input_L_Tdelay"=w470, "input_L_delayOpt"=w469, "input_T_state"=w463, "input_iSpout"=w439, "input_iTrial_relative"=w462, "input_L_T"=w441) -> ("output_LC_Event"=w461:bool, "output_LC_Laser"=w460:bool, "output_L_Tstart"=w459:u16, "output_L_Tend"=w458:u16)  [unwired: 6 in]
              n157 = call "BRig_RT__Case_Exp__State_initTrial__LC.vi"("input_L_OnOff"=w464, "input_L_Block"=w439, "input_L_Count"=w465, "input_L_Prob"=w466, "input_L_Tdelay"=w467, "input_L_delayOpt"=w468, "input_T_state"=w463, "input_iSpout"=w439, "input_iTrial_relative"=w462, "input_L_T"=w440) -> ("output_LC_Event"=w455:bool, "output_LC_Laser"=w457:bool, "output_L_Tstart"=w456:u16, "output_L_Tend"=w454:u16)  [unwired: 6 in]
            }
          }
          n158 = case shown="1" w44 {
            tunnel: w56 -> [_ w310 w332 w368]
            tunnel: w43 -> [_ w289 w311 w333]
            tunnel: w58 -> [_ w304 w326 w357]
            tunnel: w42 -> [_ w303 w325 w356]
            tunnel: [w287 w302 w314 w355] -> w71
            tunnel: [w287 w301 w314 w354] -> w70
            tunnel: [w288 w300 w313 w353] -> w66
            tunnel: [w288 w299 w313 w352] -> w64
            tunnel: [w287 w292 w324 w351] -> w68
            tunnel: [w288 w291 w323 w350] -> w62
            tunnel: [w287 w292 w322 w349] -> w69
            tunnel: [w288 w291 w321 w348] -> w60
            tunnel: w36 -> [_ w298 _ w347]
            tunnel: w35 -> [_ w297 _ w346]
            tunnel: w34 -> [_ w296 _ w345]
            tunnel: w33 -> [_ w295 _ w344]
            tunnel: w32 -> [_ w294 _ w343]
            tunnel: w31 -> [_ w293 _ w342]
            tunnel: w30 -> [_ _ w320 w341]
            tunnel: w29 -> [_ _ w319 w340]
            tunnel: w28 -> [_ _ w318 w339]
            tunnel: w27 -> [_ _ w317 w338]
            tunnel: w26 -> [_ _ w316 w337]
            tunnel: w25 -> [_ _ w315 w336]
            tunnel: w73 -> [_ w290 _ w335]
            tunnel: w72 -> [_ _ w312 w334]
            frame 0, Default {
              w288 = u16 0
              w287 = FALSE
              # "No active lasers"
            }
            frame 1 {
              w291 = u16 0
              w292 = FALSE
              # "laser1 is active"
              n159 = Index Array(array=w310, index #1=w298, index #2=w297, index #3=w296, index #4=w295, index #5=w294, index #6=w293) -> (element #1=w309:u16, element #3=w308:u16, element #4=w307:u16, element #5=w306:u16, element #6=w305:u16)  [unwired: 1 out]
              n160 = call "BRig_RT__Case_Exp__State_initTrial__LC.vi"("input_L_OnOff"=w309, "input_L_Block"=w289, "input_L_Count"=w308, "input_L_Prob"=w307, "input_L_Tdelay"=w306, "input_L_delayOpt"=w305, "input_T_state"=w304, "input_iSpout"=w289, "input_iTrial_relative"=w303, "input_L_T"=w290) -> ("output_LC_Event"=w302:bool, "output_LC_Laser"=w301:bool, "output_L_Tstart"=w300:u16, "output_L_Tend"=w299:u16)  [unwired: 6 in]
            }
            frame 2 {
              w313 = u16 0
              w314 = FALSE
              # "laser2 is active"
              n161 = Index Array(array=w332, index #1=w320, index #2=w319, index #3=w318, index #4=w317, index #5=w316, index #6=w315) -> (element #1=w327:u16, element #3=w328:u16, element #4=w329:u16, element #5=w330:u16, element #6=w331:u16)  [unwired: 1 out]
              n162 = call "BRig_RT__Case_Exp__State_initTrial__LC.vi"("input_L_OnOff"=w327, "input_L_Block"=w311, "input_L_Count"=w328, "input_L_Prob"=w329, "input_L_Tdelay"=w330, "input_L_delayOpt"=w331, "input_T_state"=w326, "input_iSpout"=w311, "input_iTrial_relative"=w325, "input_L_T"=w312) -> ("output_LC_Event"=w322:bool, "output_LC_Laser"=w324:bool, "output_L_Tstart"=w323:u16, "output_L_Tend"=w321:u16)  [unwired: 6 in]
            }
            frame 3 {
              # "laser1 and laser2 are active"
              n163 = Index Array(array=w368, index #1=w347, index #2=w346, index #3=w345, index #4=w344, index #5=w343, index #6=w342, index #7=w341, index #8=w340, index #9=w339, index #10=w338, index #11=w337, index #12=w336) -> (element #1=w367:u16, element #3=w366:u16, element #4=w365:u16, element #5=w364:u16, element #6=w363:u16, element #7=w358:u16, element #9=w359:u16, element #10=w360:u16, element #11=w361:u16, element #12=w362:u16)  [unwired: 2 out]
              n164 = call "BRig_RT__Case_Exp__State_initTrial__LC.vi"("input_L_OnOff"=w367, "input_L_Block"=w333, "input_L_Count"=w366, "input_L_Prob"=w365, "input_L_Tdelay"=w364, "input_L_delayOpt"=w363, "input_T_state"=w357, "input_iSpout"=w333, "input_iTrial_relative"=w356, "input_L_T"=w335) -> ("output_LC_Event"=w355:bool, "output_LC_Laser"=w354:bool, "output_L_Tstart"=w353:u16, "output_L_Tend"=w352:u16)  [unwired: 6 in]
              n165 = call "BRig_RT__Case_Exp__State_initTrial__LC.vi"("input_L_OnOff"=w358, "input_L_Block"=w333, "input_L_Count"=w359, "input_L_Prob"=w360, "input_L_Tdelay"=w361, "input_L_delayOpt"=w362, "input_T_state"=w357, "input_iSpout"=w333, "input_iTrial_relative"=w356, "input_L_T"=w334) -> ("output_LC_Event"=w349:bool, "output_LC_Laser"=w351:bool, "output_L_Tstart"=w350:u16, "output_L_Tend"=w348:u16)  [unwired: 6 in]
            }
          }
          n166 = call "BRig_dataCurrent_L_ENL_T_start_l1.vi"() -> ("output_L_ENL_T_start_l1"=w115:i32)  [unwired: 11 in]
          n167 = call "BRig_dataCurrent_L_ENL_T_end_l1.vi"() -> ("output_L_ENL_T_end_l1"=w113:i32)  [unwired: 11 in]
          n168 = call "BRig_dataCurrent_L_ENL_T_start_l2.vi"() -> ("output_L_T_ENL1_start_l2"=w111:i32)  [unwired: 11 in]
          n169 = call "BRig_dataCurrent_L_ENL_T_end_l2.vi"() -> ("output_L_ENL_T_end_l2"=w109:i32)  [unwired: 11 in]
          n170 = call "BRig_dataCurrent_L_ENL2_T_start_l1.vi"() -> ("output_L_ENL2_T_start_l1"=w67:i32)  [unwired: 11 in]
          n171 = call "BRig_dataCurrent_L_ENL2_T_end_l1.vi"() -> ("output_L_ENL2_T_end_l1"=w65:i32)  [unwired: 11 in]
          n172 = call "BRig_dataCurrent_L_ENL2_T_start_l2.vi"() -> ("output_L_T_ENL2_start_l2"=w63:i32)  [unwired: 11 in]
          n173 = call "BRig_dataCurrent_L_ENL2_T_end_l2.vi"() -> ("output_L_ENL2_T_end_l2"=w61:i32)  [unwired: 11 in]
          n174 = Replace Array Subset(array=w117, new element #1=w114, index #1=w115, new element #2=w112, index #2=w113, new element #3=w110, index #3=w111, new element #4=w108, index #4=w109, new element #5=w66, index #5=w67, new element #6=w64, index #6=w65, new element #7=w62, index #7=w63, new element #8=w60, index #8=w61) -> (w116:u16[])
          n175 = call "BRig_dataTrial_L_ENL_event_I_l1.vi"() -> ("output_L_ENL_event_I_l1"=w130:i32)  [unwired: 11 in]
          n176 = call "BRig_dataTrial_L_ENL_trig_I_l1.vi"() -> ("output_L_ENL_trig_I_l1"=w127:i32)  [unwired: 11 in]
          n177 = call "BRig_dataTrial_L_ENL_event_I_l2.vi"() -> ("output_L_ENL_event_I_l2"=w126:i32)  [unwired: 11 in]
          n178 = call "BRig_dataTrial_L_ENL_trig_I_l2.vi"() -> ("output_L_ENL_trig_I_l2"=w125:i32)  [unwired: 11 in]
          n179 = call "BRig_dataTrial_L_ENL2_event_I_l1.vi"() -> ("output_L_ENL2_event_I_l1"=w82:i32)  [unwired: 11 in]
          n180 = call "BRig_dataTrial_L_ENL2_trig_I_l1.vi"() -> ("output_L_ENL2_trig_I_l1"=w81:i32)  [unwired: 11 in]
          n181 = call "BRig_dataTrial_L_ENL2_event_I_l2.vi"() -> ("output_L_ENL2_event_I_l2"=w80:i32)  [unwired: 11 in]
          n182 = call "BRig_dataTrial_L_ENL2_trig_I_l2.vi"() -> ("output_L_ENL2_trig_I_l2"=w78:i32)  [unwired: 11 in]
          n183 = call "BRig_arrTrig_L_ENL_event_l1.vi"() -> ("output_L_ENL_event_l1"=w138:i32)  [unwired: 11 in]
          n184 = call "BRig_arrTrig_L_ENL_laser_l1.vi"() -> ("output_L_ENL_laserTrig_l1"=w137:i32)  [unwired: 11 in]
          n185 = call "BRig_arrTrig_L_ENL_event_l2.vi"() -> ("output_L_ENL_event_l2"=w136:i32)  [unwired: 11 in]
          n186 = call "BRig_arrTrig_L_ENL_laser_l2.vi"() -> ("output_L_ENL_laserTrig_l2"=w135:i32)  [unwired: 11 in]
          n187 = call "BRig_arrTrig_L_ENL2_event_l1.vi"() -> ("output_L_ENL2_event_l1"=w90:i32)  [unwired: 11 in]
          n188 = call "BRig_arrTrig_L_ENL2_laser_l1.vi"() -> ("output_L_ENL2_laserTrig_l1"=w89:i32)  [unwired: 11 in]
          n189 = call "BRig_arrTrig_L_ENL2_event_l2.vi"() -> ("output_L_ENL2_event_l2"=w88:i32)  [unwired: 11 in]
          n190 = call "BRig_arrTrig_L_ENL2_laser_l2.vi"() -> ("output_L_ENL2_laserTrig_l2"=w87:i32)  [unwired: 11 in]
          n191 = Boolean To (0,1)(Boolean=w129) -> (0, 1=w134:i16)
          n192 = Boolean To (0,1)(Boolean=w123) -> (0, 1=w133:i16)
          n193 = Boolean To (0,1)(Boolean=w121) -> (0, 1=w131:i16)
          n194 = Boolean To (0,1)(Boolean=w119) -> (0, 1=w132:i16)
          n195 = Boolean To (0,1)(Boolean=w71) -> (0, 1=w86:i16)
          n196 = Boolean To (0,1)(Boolean=w70) -> (0, 1=w85:i16)
          n197 = Boolean To (0,1)(Boolean=w69) -> (0, 1=w83:i16)
          n198 = Boolean To (0,1)(Boolean=w68) -> (0, 1=w84:i16)
          n199 = Replace Array Subset(array=w140, new element #1=w129, index #1=w138, new element #2=w123, index #2=w137, new element #3=w121, index #3=w136, new element #4=w119, index #4=w135, new element #5=w71, index #5=w90, new element #6=w70, index #6=w89, new element #7=w69, index #7=w88, new element #8=w68, index #8=w87) -> (w139:bool[])
          n200 = To Unsigned Word Integer(number=w134) -> (unsigned 16bit integer=w128:u16)
          n201 = To Unsigned Word Integer(number=w133) -> (unsigned 16bit integer=w124:u16)
          n202 = To Unsigned Word Integer(number=w131) -> (unsigned 16bit integer=w122:u16)
          n203 = To Unsigned Word Integer(number=w132) -> (unsigned 16bit integer=w120:u16)
          n204 = To Unsigned Word Integer(number=w86) -> (unsigned 16bit integer=w77:u16)
          n205 = To Unsigned Word Integer(number=w85) -> (unsigned 16bit integer=w76:u16)
          n206 = To Unsigned Word Integer(number=w83) -> (unsigned 16bit integer=w75:u16)
          n207 = To Unsigned Word Integer(number=w84) -> (unsigned 16bit integer=w74:u16)
          n208 = Replace Array Subset(array=w57, new element #1=w128, index (row) #1=w79, index (col) #1=w130, new element #2=w124, index (row) #2=w79, index (col) #2=w127, new element #3=w122, index (row) #3=w79, index (col) #3=w126, new element #4=w120, index (row) #4=w79, index (col) #4=w125, new element #5=w77, index (row) #5=w79, index (col) #5=w82, new element #6=w76, index (row) #6=w79, index (col) #6=w81, new element #7=w75, index (row) #7=w79, index (col) #7=w80, new element #8=w74, index (row) #8=w79, index (col) #8=w78) -> (w118:u16[][])
        }
        frame False {
          w478 = u16 1
          w479 = u16 0
          w480 = u16 2 ("input_sState_start")
          w528 = 0
          # "dataLC_ENL2_ [ ]\nnot used anymore"
          # "Need to force block condition to pass\nby setting iSpout = Block\nwhere Block is Block parameter\nfor both l1 and l2, and Reward and Wrong"
          # "Record laser timing"
          # "Calculate laser timing"
          # "Total Time (ENL2)"
          # "Total Time (ENL)"
          # "iTrial\nrelative"
          # "Total Time (Laser 2)"
          # "Total Time (Laser 1)"
          # "laser timing case (ENL2)"
          # "Determine case for\ncalculating laser timing"
          # "2) Get relative iTrial"
          # "1) If Trial Start State = PostReward,\nThen check LC_ENL_nReward"
          # "laser2 active (ENL2)?"
          # "laser1 active (ENL2)?"
          # "laser2 active (ENL)?"
          # "laser1 active (ENL)?"
          # "1) If Trial Start State = PostReward,\nThen check LC_ENL_nReward\n\n2) Get relative iTrial"
          # "Gather variables"
          # "Last trial's\niReward\n(0 = not reward)"
          # "idx dataTrial"
          # "Total Time (ENL2)"
          # "Total Time (ENL)"
          # "Have ENL2?"
          # "Total Time (Laser 2)"
          # "Total Time (Laser 1)"
          # "Calculate settings for ENL2"
          # "Calculate settings for ENL"
          # "Set laser settings for ENL and ENL2"
          # "iTrial\nrelative"
          # "laser timing case (ENL)"
          # "Trial start state\n0 (unknown)\n1 (first)\n2 (PreReward)\n3 (PostReward)"
          # "laser2 active?"
          # "laser1 active?"
          n209 = call "BRig_dataCurrent_LaserSwitch_l1.vi"() -> ("output_LaserSwitch_l1"=w597:i32)  [unwired: 11 in]
          n210 = call "BRig_dataCurrent_LaserSwitch_l2.vi"() -> ("output_LaserSwitch_l2"=w596:i32)  [unwired: 11 in]
          n211 = call "BRig_dataExp_L_Ttotal_l1.vi"() -> ("output_L_Ttotal_l1"=w543:i32)  [unwired: 11 in]
          n212 = call "BRig_dataExp_L_Ttotal_l2.vi"() -> ("output_L_Ttotal_l2"=w544:i32)  [unwired: 11 in]
          n213 = call "BRig_dataTrial_T_ENL.vi"() -> ("output_T_ENL"=w541:i32)  [unwired: 11 in]
          n214 = call "BRig_dataTrial_T_ENL2.vi"() -> ("output_T_ENL2"=w540:i32)  [unwired: 11 in]
          n215 = Index Array(array=w566, index #1=w597, index #2=w596) -> (element #1=w595:u16, element #2=w594:u16)
          n216 = Index Array(array=w542, index #1=w543, index #2=w544) -> (element #1=w522:u16, element #2=w521:u16)
          n217 = Index Array(array=w494, index (row) #1=w528, index (col) #1=w541, index (row) #2=w528, index (col) #2=w540) -> (element #1=w496:u16, element #2=w495:u16)
          n218 = Not Equal To 0?(x=w595) -> (x != 0?=w491:bool)
          n219 = Not Equal To 0?(x=w594) -> (x != 0?=w492:bool)
          n220 = case shown="0" w478 {
            tunnel: u16 0 -> [_ _ w612]
            tunnel: w493 -> [_ _ w613]
            tunnel: w492 -> [_ w602 w605]
            tunnel: w491 -> [_ w603 w606]
            tunnel: w477 -> [_ w601 w604]
            tunnel: [w598 w603 w611] -> w490
            tunnel: [w598 w602 w610] -> w489
            tunnel: [w598 w600 w609] -> w484
            tunnel: [w598 w599 w608] -> w483
            frame 0 {
              w598 = FALSE
            }
            frame 1, Default {
              n221 = And(x=w601, y=w603) -> (x .and. y?=w600:bool)
              n222 = And(x=w602, y=w601) -> (x .and. y?=w599:bool)
            }
            frame 3 {
              w618 = i16 0 ("f")
              n223 = Boolean To (0,1)(Boolean=w606) -> (0, 1=w616:i16)
              n224 = Select(t=i16 2, s=w605, f=w618) -> (s? t:f=w617:i16)
              n225 = Select(t=i16 4, s=w604, f=w618) -> (s? t:f=w615:i16)
              n226 = Compound Arithmetic op=ADD(w616, w617, w615) -> (w614:i16)
              n227 = case shown="7" w614 {
                tunnel: w613 -> [_ w625 w636 w648 _ w675 w698 w721]
                tunnel: w612 -> [_ w624 w635 w647 _ w671 w694 w706]
                tunnel: [w621 w623 w633 w646 w663 w670 w691 w705] -> w611
                tunnel: [w621 w622 w634 w645 w663 w668 w693 w704] -> w610
                tunnel: [w621 w622 w633 w644 w663 w669 w691 w703] -> w609
                tunnel: [w621 w622 w633 w644 w663 w668 w692 w702] -> w608
                tunnel: FALSE -> [w621 w622 w633 w644 w663 w668 w691 _]
                frame 0, Default {
                }
                frame 1 {
                  n228 = call "BRig_dataLC_ENL_PostR_nRew1_l1.vi"() -> ("output_ENL_PostR_nRew1_l1"=w632:i32)  [unwired: 11 in]
                  n229 = call "BRig_dataLC_ENL_PostR_nRew2_l1.vi"() -> ("output_ENL_PostR_nRew2_l1"=w631:i32)  [unwired: 11 in]
                  n230 = Index Array(array=w625, index #1=w632, index #2=w631) -> (element #1=w627:u16, element #2=w626:u16)
                  n231 = Equal To 0?(x=w627) -> (x = 0?=w628:bool)
                  n232 = Equal?(x=w627, y=w624) -> (x = y?=w629:bool)
                  n233 = Equal?(x=w626, y=w624) -> (x = y?=w630:bool)
                  n234 = Compound Arithmetic op=OR(w628, w629, w630) -> (w623:bool)
                }
                frame 2 {
                  n235 = call "BRig_dataLC_ENL_PostR_nRew1_l2.vi"() -> ("output_ENL_PostR_nRew1_l2"=w643:i32)  [unwired: 11 in]
                  n236 = call "BRig_dataLC_ENL_PostR_nRew2_l2.vi"() -> ("output_ENL_PostR_nRew2_l2"=w642:i32)  [unwired: 11 in]
                  n237 = Index Array(array=w636, index #1=w643, index #2=w642) -> (element #1=w637:u16, element #2=w638:u16)
                  n238 = Equal To 0?(x=w637) -> (x = 0?=w640:bool)
                  n239 = Equal?(x=w637, y=w635) -> (x = y?=w639:bool)
                  n240 = Equal?(x=w638, y=w635) -> (x = y?=w641:bool)
                  n241 = Compound Arithmetic op=OR(w640, w639, w641) -> (w634:bool)
                }
                frame 3 {
                  n242 = call "BRig_dataLC_ENL_PostR_nRew1_l1.vi"() -> ("output_ENL_PostR_nRew1_l1"=w662:i32)  [unwired: 11 in]
                  n243 = call "BRig_dataLC_ENL_PostR_nRew2_l1.vi"() -> ("output_ENL_PostR_nRew2_l1"=w661:i32)  [unwired: 11 in]
                  n244 = call "BRig_dataLC_ENL_PostR_nRew1_l2.vi"() -> ("output_ENL_PostR_nRew1_l2"=w660:i32)  [unwired: 11 in]
                  n245 = call "BRig_dataLC_ENL_PostR_nRew2_l2.vi"() -> ("output_ENL_PostR_nRew2_l2"=w659:i32)  [unwired: 11 in]
                  n246 = Index Array(array=w648, index #1=w662, index #2=w661, index #3=w660, index #4=w659) -> (element #1=w652:u16, element #2=w651:u16, element #3=w649:u16, element #4=w650:u16)
                  n247 = Equal To 0?(x=w652) -> (x = 0?=w653:bool)
                  n248 = Equal?(x=w652, y=w647) -> (x = y?=w654:bool)
                  n249 = Equal?(x=w651, y=w647) -> (x = y?=w655:bool)
                  n250 = Equal To 0?(x=w649) -> (x = 0?=w657:bool)
                  n251 = Equal?(x=w649, y=w647) -> (x = y?=w656:bool)
                  n252 = Equal?(x=w650, y=w647) -> (x = y?=w658:bool)
                  n253 = Compound Arithmetic op=OR(w653, w654, w655) -> (w646:bool)
                  n254 = Compound Arithmetic op=OR(w657, w656, w658) -> (w645:bool)
                }
                frame 4 {
                }
                frame 5 {
                  n255 = call "BRig_dataLC_ENL_PostR_nRew1_l1.vi"() -> ("output_ENL_PostR_nRew1_l1"=w682:i32)  [unwired: 11 in]
                  n256 = call "BRig_dataLC_ENL_PostR_nRew2_l1.vi"() -> ("output_ENL_PostR_nRew2_l1"=w681:i32)  [unwired: 11 in]
                  n257 = call "BRig_dataLC_ENL2_PostR_nRew1_l1.vi"() -> ("output_ENL2_PostR_nRew1_l1"=w667:i32)  [unwired: 11 in]
                  n258 = call "BRig_dataLC_ENL2_PostR_nRew2_l1.vi"() -> ("output_ENL2_PostR_nRew2_l1"=w666:i32)  [unwired: 11 in]
                  n259 = Index Array(array=w675, index #1=w682, index #2=w681, index #3=w667, index #4=w666) -> (element #1=w677:u16, element #2=w676:u16, element #3=w665:u16, element #4=w664:u16)
                  n260 = Equal To 0?(x=w677) -> (x = 0?=w678:bool)
                  n261 = Equal?(x=w677, y=w671) -> (x = y?=w679:bool)
                  n262 = Equal?(x=w676, y=w671) -> (x = y?=w680:bool)
                  n263 = Equal To 0?(x=w665) -> (x = 0?=w674:bool)
                  n264 = Equal?(x=w665, y=w671) -> (x = y?=w673:bool)
                  n265 = Equal?(x=w664, y=w671) -> (x = y?=w672:bool)
                  n266 = Compound Arithmetic op=OR(w678, w679, w680) -> (w670:bool)
                  n267 = Compound Arithmetic op=OR(w674, w673, w672) -> (w669:bool)
                }
                frame 6 {
                  n268 = call "BRig_dataLC_ENL_PostR_nRew1_l2.vi"() -> ("output_ENL_PostR_nRew1_l2"=w690:i32)  [unwired: 11 in]
                  n269 = call "BRig_dataLC_ENL_PostR_nRew2_l2.vi"() -> ("output_ENL_PostR_nRew2_l2"=w689:i32)  [unwired: 11 in]
                  n270 = call "BRig_dataLC_ENL2_PostR_nRew1_l2.vi"() -> ("output_ENL2_PostR_nRew1_l2"=w686:i32)  [unwired: 11 in]
                  n271 = call "BRig_dataLC_ENL2_PostR_nRew2_l2.vi"() -> ("output_ENL2_PostR_nRew2_l2"=w685:i32)  [unwired: 11 in]
                  n272 = Index Array(array=w698, index #1=w690, index #2=w689, index #3=w686, index #4=w685) -> (element #1=w688:u16, element #2=w687:u16, element #3=w684:u16, element #4=w683:u16)
                  n273 = Equal To 0?(x=w688) -> (x = 0?=w700:bool)
                  n274 = Equal?(x=w688, y=w694) -> (x = y?=w699:bool)
                  n275 = Equal?(x=w687, y=w694) -> (x = y?=w701:bool)
                  n276 = Equal To 0?(x=w684) -> (x = 0?=w696:bool)
                  n277 = Equal?(x=w684, y=w694) -> (x = y?=w697:bool)
                  n278 = Equal?(x=w683, y=w694) -> (x = y?=w695:bool)
                  n279 = Compound Arithmetic op=OR(w700, w699, w701) -> (w693:bool)
                  n280 = Compound Arithmetic op=OR(w696, w697, w695) -> (w692:bool)
                }
                frame 7 {
                  n281 = call "BRig_dataLC_ENL_PostR_nRew1_l1.vi"() -> ("output_ENL_PostR_nRew1_l1"=w735:i32)  [unwired: 11 in]
                  n282 = call "BRig_dataLC_ENL_PostR_nRew2_l1.vi"() -> ("output_ENL_PostR_nRew2_l1"=w734:i32)  [unwired: 11 in]
                  n283 = call "BRig_dataLC_ENL_PostR_nRew1_l2.vi"() -> ("output_ENL_PostR_nRew1_l2"=w733:i32)  [unwired: 11 in]
                  n284 = call "BRig_dataLC_ENL_PostR_nRew2_l2.vi"() -> ("output_ENL_PostR_nRew2_l2"=w732:i32)  [unwired: 11 in]
                  n285 = call "BRig_dataLC_ENL2_PostR_nRew1_l1.vi"() -> ("output_ENL2_PostR_nRew1_l1"=w720:i32)  [unwired: 11 in]
                  n286 = call "BRig_dataLC_ENL2_PostR_nRew2_l1.vi"() -> ("output_ENL2_PostR_nRew2_l1"=w719:i32)  [unwired: 11 in]
                  n287 = call "BRig_dataLC_ENL2_PostR_nRew1_l2.vi"() -> ("output_ENL2_PostR_nRew1_l2"=w718:i32)  [unwired: 11 in]
                  n288 = call "BRig_dataLC_ENL2_PostR_nRew2_l2.vi"() -> ("output_ENL2_PostR_nRew2_l2"=w717:i32)  [unwired: 11 in]
                  n289 = Index Array(array=w721, index #1=w735, index #2=w734, index #3=w733, index #4=w732, index #5=w720, index #6=w719, index #7=w718, index #8=w717) -> (element #1=w725:u16, element #2=w724:u16, element #3=w722:u16, element #4=w723:u16, element #5=w710:u16, element #6=w709:u16, element #7=w707:u16, element #8=w708:u16)
                  n290 = Equal To 0?(x=w725) -> (x = 0?=w726:bool)
                  n291 = Equal?(x=w725, y=w706) -> (x = y?=w727:bool)
                  n292 = Equal?(x=w724, y=w706) -> (x = y?=w728:bool)
                  n293 = Equal To 0?(x=w722) -> (x = 0?=w730:bool)
                  n294 = Equal?(x=w722, y=w706) -> (x = y?=w729:bool)
                  n295 = Equal?(x=w723, y=w706) -> (x = y?=w731:bool)
                  n296 = Equal To 0?(x=w710) -> (x = 0?=w716:bool)
                  n297 = Equal?(x=w710, y=w706) -> (x = y?=w715:bool)
                  n298 = Equal?(x=w709, y=w706) -> (x = y?=w714:bool)
                  n299 = Equal To 0?(x=w707) -> (x = 0?=w712:bool)
                  n300 = Equal?(x=w707, y=w706) -> (x = y?=w713:bool)
                  n301 = Equal?(x=w708, y=w706) -> (x = y?=w711:bool)
                  n302 = Compound Arithmetic op=OR(w726, w727, w728) -> (w705:bool)
                  n303 = Compound Arithmetic op=OR(w730, w729, w731) -> (w704:bool)
                  n304 = Compound Arithmetic op=OR(w716, w715, w714) -> (w703:bool)
                  n305 = Compound Arithmetic op=OR(w712, w713, w711) -> (w702:bool)
                }
              }
            }
          }
          n306 = case shown="1, Default" w478 {
            tunnel: [w865 w877 w889] -> w556
            tunnel: [w864 w876 w878] -> w555
            tunnel: [w863 w875 w879] -> w554
            tunnel: [w862 w874 w880] -> w553
            tunnel: [w861 w873 w881] -> w552
            tunnel: [w860 w872 w882] -> w551
            tunnel: [w859 w871 w888] -> w550
            tunnel: [w858 w870 w887] -> w549
            tunnel: [w857 w869 w886] -> w548
            tunnel: [w856 w868 w885] -> w547
            tunnel: [w855 w867 w884] -> w546
            tunnel: [w854 w866 w883] -> w545
            frame 1, Default {
              n307 = call "BRig_dataLC_ENL_First_OnOff_l1.vi"() -> ("output_ENL_First_OnOff"=w865:i32)  [unwired: 11 in]
              n308 = call "BRig_dataLC_ENL_First_Block_l1.vi"() -> ("output_ENL_First_Block"=w864:i32)  [unwired: 11 in]
              n309 = call "BRig_dataLC_ENL_First_Count_l1.vi"() -> ("output_ENL_First_Count"=w863:i32)  [unwired: 11 in]
              n310 = call "BRig_dataLC_ENL_First_Prob_l1.vi"() -> ("output_ENL_First_Prob"=w862:i32)  [unwired: 11 in]
              n311 = call "BRig_dataLC_ENL_First_Delay_l1.vi"() -> ("output_ENL_First_Delay"=w861:i32)  [unwired: 11 in]
              n312 = call "BRig_dataLC_ENL_First_DelayOpt_l1.vi"() -> ("output_ENL_First_DelayOpt"=w860:i32)  [unwired: 11 in]
              n313 = call "BRig_dataLC_ENL_First_OnOff_l2.vi"() -> ("output_ENL_First_OnOff_l2"=w859:i32)  [unwired: 11 in]
              n314 = call "BRig_dataLC_ENL_First_Block_l2.vi"() -> ("output_ENL_First_Block_l2"=w858:i32)  [unwired: 11 in]
              n315 = call "BRig_dataLC_ENL_First_Count_l2.vi"() -> ("output_ENL_First_Count_l2"=w857:i32)  [unwired: 11 in]
              n316 = call "BRig_dataLC_ENL_First_Prob_l2.vi"() -> ("output_ENL_First_Prob_l2"=w856:i32)  [unwired: 11 in]
              n317 = call "BRig_dataLC_ENL_First_Delay_l2.vi"() -> ("output_ENL_First_Delay_l2"=w855:i32)  [unwired: 11 in]
              n318 = call "BRig_dataLC_ENL_First_DelayOpt_l2.vi"() -> ("output_ENL_First_DelayOpt_l2"=w854:i32)  [unwired: 11 in]
            }
            frame 2 {
              n319 = call "BRig_dataLC_ENL_PreR_OnOff_l1.vi"() -> ("output_ENL_PreR_OnOff"=w877:i32)  [unwired: 11 in]
              n320 = call "BRig_dataLC_ENL_PreR_Block_l1.vi"() -> ("output_ENL_PreR_Block"=w876:i32)  [unwired: 11 in]
              n321 = call "BRig_dataLC_ENL_PreR_Count_l1.vi"() -> ("output_ENL_PreR_Count"=w875:i32)  [unwired: 11 in]
              n322 = call "BRig_dataLC_ENL_PreR_Prob_l1.vi"() -> ("output_ENL_PreR_Prob"=w874:i32)  [unwired: 11 in]
              n323 = call "BRig_dataLC_ENL_PreR_Delay_l1.vi"() -> ("output_ENL_PreR_Delay"=w873:i32)  [unwired: 11 in]
              n324 = call "BRig_dataLC_ENL_PreR_DelayOpt_l1.vi"() -> ("output_ENL_PreR_DelayOpt"=w872:i32)  [unwired: 11 in]
              n325 = call "BRig_dataLC_ENL_PreR_OnOff_l2.vi"() -> ("output_ENL_PreR_OnOff_l2"=w871:i32)  [unwired: 11 in]
              n326 = call "BRig_dataLC_ENL_PreR_Block_l2.vi"() -> ("output_ENL_PreR_Block_l2"=w870:i32)  [unwired: 11 in]
              n327 = call "BRig_dataLC_ENL_PreR_Count_l2.vi"() -> ("output_ENL_PreR_Count_l2"=w869:i32)  [unwired: 11 in]
              n328 = call "BRig_dataLC_ENL_PreR_Prob_l2.vi"() -> ("output_ENL_PreR_Prob_l2"=w868:i32)  [unwired: 11 in]
              n329 = call "BRig_dataLC_ENL_PreR_Delay_l2.vi"() -> ("output_ENL_PreR_Delay_l2"=w867:i32)  [unwired: 11 in]
              n330 = call "BRig_dataLC_ENL_PreR_DelayOpt_l2.vi"() -> ("output_ENL_PreR_DelayOpt_l2"=w866:i32)  [unwired: 11 in]
            }
            frame 3 {
              n331 = call "BRig_dataLC_ENL_PostR_OnOff_l1.vi"() -> ("output_ENL_PostR_OnOff"=w889:i32)  [unwired: 11 in]
              n332 = call "BRig_dataLC_ENL_PostR_Block_l1.vi"() -> ("output_ENL_PostR_Block"=w878:i32)  [unwired: 11 in]
              n333 = call "BRig_dataLC_ENL_PostR_Count_l1.vi"() -> ("output_ENL_PostR_Count"=w879:i32)  [unwired: 11 in]
              n334 = call "BRig_dataLC_ENL_PostR_Prob_l1.vi"() -> ("output_ENL_PostR_Prob"=w880:i32)  [unwired: 11 in]
              n335 = call "BRig_dataLC_ENL_PostR_Delay_l1.vi"() -> ("output_ENL_PostR_Delay"=w881:i32)  [unwired: 11 in]
              n336 = call "BRig_dataLC_ENL_PostR_DelayOpt_l1.vi"() -> ("output_ENL_PostR_DelayOpt"=w882:i32)  [unwired: 11 in]
              n337 = call "BRig_dataLC_ENL_PostR_OnOff_l2.vi"() -> ("output_ENL_PostR_OnOff_l2"=w888:i32)  [unwired: 11 in]
              n338 = call "BRig_dataLC_ENL_PostR_Block_l2.vi"() -> ("output_ENL_PostR_Block_l2"=w887:i32)  [unwired: 11 in]
              n339 = call "BRig_dataLC_ENL_PostR_Count_l2.vi"() -> ("output_ENL_PostR_Count_l2"=w886:i32)  [unwired: 11 in]
              n340 = call "BRig_dataLC_ENL_PostR_Prob_l2.vi"() -> ("output_ENL_PostR_Prob_l2"=w885:i32)  [unwired: 11 in]
              n341 = call "BRig_dataLC_ENL_PostR_Delay_l2.vi"() -> ("output_ENL_PostR_Delay_l2"=w884:i32)  [unwired: 11 in]
              n342 = call "BRig_dataLC_ENL_PostR_DelayOpt_l2.vi"() -> ("output_ENL_PostR_DelayOpt_l2"=w883:i32)  [unwired: 11 in]
            }
          }
          n343 = case shown="1, Default" w478 {
            tunnel: [w747 w759 w771] -> w520
            tunnel: [w746 w758 w770] -> w519
            tunnel: [w745 w757 w769] -> w518
            tunnel: [w744 w756 w768] -> w517
            tunnel: [w743 w755 w767] -> w516
            tunnel: [w742 w754 w766] -> w515
            tunnel: [w741 w753 w765] -> w514
            tunnel: [w740 w752 w764] -> w513
            tunnel: [w739 w751 w763] -> w512
            tunnel: [w738 w750 w762] -> w511
            tunnel: [w737 w749 w761] -> w510
            tunnel: [w736 w748 w760] -> w509
            frame 1, Default {
              n344 = call "BRig_dataLC_ENL2_First_OnOff_l1.vi"() -> ("output_ENL2_First_OnOff"=w747:i32)  [unwired: 11 in]
              n345 = call "BRig_dataLC_ENL2_First_Block_l1.vi"() -> ("output_ENL2_First_Block"=w746:i32)  [unwired: 11 in]
              n346 = call "BRig_dataLC_ENL2_First_Count_l1.vi"() -> ("output_ENL2_First_Count"=w745:i32)  [unwired: 11 in]
              n347 = call "BRig_dataLC_ENL2_First_Prob_l1.vi"() -> ("output_ENL2_First_Prob"=w744:i32)  [unwired: 11 in]
              n348 = call "BRig_dataLC_ENL2_First_Delay_l1.vi"() -> ("output_ENL2_First_Delay"=w743:i32)  [unwired: 11 in]
              n349 = call "BRig_dataLC_ENL2_First_DelayOpt_l1.vi"() -> ("output_ENL2_First_DelayOpt"=w742:i32)  [unwired: 11 in]
              n350 = call "BRig_dataLC_ENL2_First_OnOff_l2.vi"() -> ("output_ENL2_First_OnOff_l2"=w741:i32)  [unwired: 11 in]
              n351 = call "BRig_dataLC_ENL2_First_Block_l2.vi"() -> ("output_ENL2_First_Block_l2"=w740:i32)  [unwired: 11 in]
              n352 = call "BRig_dataLC_ENL2_First_Count_l2.vi"() -> ("output_ENL2_First_Count_l2"=w739:i32)  [unwired: 11 in]
              n353 = call "BRig_dataLC_ENL2_First_Prob_l2.vi"() -> ("output_ENL2_First_Prob_l2"=w738:i32)  [unwired: 11 in]
              n354 = call "BRig_dataLC_ENL2_First_Delay_l2.vi"() -> ("output_ENL2_First_Delay_l2"=w737:i32)  [unwired: 11 in]
              n355 = call "BRig_dataLC_ENL2_First_DelayOpt_l2.vi"() -> ("output_ENL2_First_DelayOpt_l2"=w736:i32)  [unwired: 11 in]
            }
            frame 2 {
              n356 = call "BRig_dataLC_ENL2_PreR_OnOff_l1.vi"() -> ("output_ENL2_PreR_OnOff"=w759:i32)  [unwired: 11 in]
              n357 = call "BRig_dataLC_ENL2_PreR_Block_l1.vi"() -> ("output_ENL2_PreR_Block"=w758:i32)  [unwired: 11 in]
              n358 = call "BRig_dataLC_ENL2_PreR_Count_l1.vi"() -> ("output_ENL2_PreR_Count"=w757:i32)  [unwired: 11 in]
              n359 = call "BRig_dataLC_ENL2_PreR_Prob_l1.vi"() -> ("output_ENL2_PreR_Prob"=w756:i32)  [unwired: 11 in]
              n360 = call "BRig_dataLC_ENL2_PreR_Delay_l1.vi"() -> ("output_ENL2_PreR_Delay"=w755:i32)  [unwired: 11 in]
              n361 = call "BRig_dataLC_ENL2_PreR_DelayOpt_l1.vi"() -> ("output_ENL2_PreR_DelayOpt"=w754:i32)  [unwired: 11 in]
              n362 = call "BRig_dataLC_ENL2_PreR_OnOff_l2.vi"() -> ("output_ENL2_PreR_OnOff_l2"=w753:i32)  [unwired: 11 in]
              n363 = call "BRig_dataLC_ENL2_PreR_Block_l2.vi"() -> ("output_ENL2_PreR_Block_l2"=w752:i32)  [unwired: 11 in]
              n364 = call "BRig_dataLC_ENL2_PreR_Count_l2.vi"() -> ("output_ENL2_PreR_Count_l2"=w751:i32)  [unwired: 11 in]
              n365 = call "BRig_dataLC_ENL2_PreR_Prob_l2.vi"() -> ("output_ENL2_PreR_Prob_l2"=w750:i32)  [unwired: 11 in]
              n366 = call "BRig_dataLC_ENL2_PreR_Delay_l2.vi"() -> ("output_ENL2_PreR_Delay_l2"=w749:i32)  [unwired: 11 in]
              n367 = call "BRig_dataLC_ENL2_PreR_DelayOpt_l2.vi"() -> ("output_ENL2_PreR_DelayOpt_l2"=w748:i32)  [unwired: 11 in]
            }
            frame 3 {
              n368 = call "BRig_dataLC_ENL2_PostR_OnOff_l1.vi"() -> ("output_ENL2_PostR_OnOff"=w771:i32)  [unwired: 11 in]
              n369 = call "BRig_dataLC_ENL2_PostR_Block_l1.vi"() -> ("output_ENL2_PostR_Block"=w770:i32)  [unwired: 11 in]
              n370 = call "BRig_dataLC_ENL2_PostR_Count_l1.vi"() -> ("output_ENL2_PostR_Count"=w769:i32)  [unwired: 11 in]
              n371 = call "BRig_dataLC_ENL2_PostR_Prob_l1.vi"() -> ("output_ENL2_PostR_Prob"=w768:i32)  [unwired: 11 in]
              n372 = call "BRig_dataLC_ENL2_PostR_Delay_l1.vi"() -> ("output_ENL2_PostR_Delay"=w767:i32)  [unwired: 11 in]
              n373 = call "BRig_dataLC_ENL2_PostR_DelayOpt_l1.vi"() -> ("output_ENL2_PostR_DelayOpt"=w766:i32)  [unwired: 11 in]
              n374 = call "BRig_dataLC_ENL2_PostR_OnOff_l2.vi"() -> ("output_ENL2_PostR_OnOff_l2"=w765:i32)  [unwired: 11 in]
              n375 = call "BRig_dataLC_ENL2_PostR_Block_l2.vi"() -> ("output_ENL2_PostR_Block_l2"=w764:i32)  [unwired: 11 in]
              n376 = call "BRig_dataLC_ENL2_PostR_Count_l2.vi"() -> ("output_ENL2_PostR_Count_l2"=w763:i32)  [unwired: 11 in]
              n377 = call "BRig_dataLC_ENL2_PostR_Prob_l2.vi"() -> ("output_ENL2_PostR_Prob_l2"=w762:i32)  [unwired: 11 in]
              n378 = call "BRig_dataLC_ENL2_PostR_Delay_l2.vi"() -> ("output_ENL2_PostR_Delay_l2"=w761:i32)  [unwired: 11 in]
              n379 = call "BRig_dataLC_ENL2_PostR_DelayOpt_l2.vi"() -> ("output_ENL2_PostR_DelayOpt_l2"=w760:i32)  [unwired: 11 in]
            }
          }
          n380 = Boolean To (0,1)(Boolean=w490) -> (0, 1=w591:i16)
          n381 = Boolean To (0,1)(Boolean=w484) -> (0, 1=w487:i16)
          n382 = Select(t=i16 2, s=w489, f=i16 0) -> (s? t:f=w592:i16)
          n383 = Select(t=i16 2, s=w483, f=i16 0) -> (s? t:f=w486:i16)
          n384 = Add(x=w591, y=w592) -> (x+y=w482:i16)
          n385 = Add(x=w487, y=w486) -> (x+y=w481:i16)
          n386 = case shown="1" w482 {
            tunnel: w493 -> [_ w913 w935 w972]
            tunnel: w480 -> [_ w892 w914 w936]
            tunnel: w496 -> [_ w907 w929 w960]
            tunnel: w479 -> [_ w906 w928 w959]
            tunnel: [w890 w905 w917 w958] -> w578
            tunnel: [w890 w904 w917 w957] -> w572
            tunnel: [w891 w903 w916 w956] -> w563
            tunnel: [w891 w902 w916 w955] -> w561
            tunnel: [w890 w895 w927 w954] -> w568
            tunnel: [w891 w894 w926 w953] -> w559
            tunnel: [w890 w895 w925 w952] -> w570
            tunnel: [w891 w894 w924 w951] -> w557
            tunnel: w556 -> [_ w901 _ w950]
            tunnel: w555 -> [_ w900 _ w949]
            tunnel: w554 -> [_ w899 _ w948]
            tunnel: w553 -> [_ w898 _ w947]
            tunnel: w552 -> [_ w897 _ w946]
            tunnel: w551 -> [_ w896 _ w945]
            tunnel: w550 -> [_ _ w923 w944]
            tunnel: w549 -> [_ _ w922 w943]
            tunnel: w548 -> [_ _ w921 w942]
            tunnel: w547 -> [_ _ w920 w941]
            tunnel: w546 -> [_ _ w919 w940]
            tunnel: w545 -> [_ _ w918 w939]
            tunnel: w522 -> [_ w893 _ w938]
            tunnel: w521 -> [_ _ w915 w937]
            frame 0, Default {
              w891 = u16 0
              w890 = FALSE
              # "No active lasers"
            }
            frame 1 {
              w894 = u16 0
              w895 = FALSE
              # "laser1 is active"
              n387 = Index Array(array=w913, index #1=w901, index #2=w900, index #3=w899, index #4=w898, index #5=w897, index #6=w896) -> (element #1=w912:u16, element #3=w911:u16, element #4=w910:u16, element #5=w909:u16, element #6=w908:u16)  [unwired: 1 out]
              n388 = call "BRig_RT__Case_Exp__State_initTrial__LC.vi"("input_L_OnOff"=w912, "input_L_Block"=w892, "input_L_Count"=w911, "input_L_Prob"=w910, "input_L_Tdelay"=w909, "input_L_delayOpt"=w908, "input_T_state"=w907, "input_iSpout"=w892, "input_iTrial_relative"=w906, "input_L_T"=w893) -> ("output_LC_Event"=w905:bool, "output_LC_Laser"=w904:bool, "output_L_Tstart"=w903:u16, "output_L_Tend"=w902:u16)  [unwired: 6 in]
            }
            frame 2 {
              w916 = u16 0
              w917 = FALSE
              # "laser2 is active"
              n389 = Index Array(array=w935, index #1=w923, index #2=w922, index #3=w921, index #4=w920, index #5=w919, index #6=w918) -> (element #1=w930:u16, element #3=w931:u16, element #4=w932:u16, element #5=w933:u16, element #6=w934:u16)  [unwired: 1 out]
              n390 = call "BRig_RT__Case_Exp__State_initTrial__LC.vi"("input_L_OnOff"=w930, "input_L_Block"=w914, "input_L_Count"=w931, "input_L_Prob"=w932, "input_L_Tdelay"=w933, "input_L_delayOpt"=w934, "input_T_state"=w929, "input_iSpout"=w914, "input_iTrial_relative"=w928, "input_L_T"=w915) -> ("output_LC_Event"=w925:bool, "output_LC_Laser"=w927:bool, "output_L_Tstart"=w926:u16, "output_L_Tend"=w924:u16)  [unwired: 6 in]
            }
            frame 3 {
              # "laser1 and laser2 are active"
              n391 = Index Array(array=w972, index #1=w950, index #2=w949, index #3=w948, index #4=w947, index #5=w946, index #6=w945, index #7=w944, index #8=w943, index #9=w942, index #10=w941, index #11=w940, index #12=w939) -> (element #1=w971:u16, element #2=w970:u16, element #3=w969:u16, element #4=w968:u16, element #5=w967:u16, element #6=w966:u16, element #7=w961:u16, element #9=w962:u16, element #10=w963:u16, element #11=w964:u16, element #12=w965:u16)  [unwired: 1 out]
              n392 = call "BRig_RT__Case_Exp__State_initTrial__LC.vi"("input_L_OnOff"=w971, "input_L_Block"=w970, "input_L_Count"=w969, "input_L_Prob"=w968, "input_L_Tdelay"=w967, "input_L_delayOpt"=w966, "input_T_state"=w960, "input_iSpout"=w936, "input_iTrial_relative"=w959, "input_L_T"=w938) -> ("output_LC_Event"=w958:bool, "output_LC_Laser"=w957:bool, "output_L_Tstart"=w956:u16, "output_L_Tend"=w955:u16)  [unwired: 6 in]
              n393 = call "BRig_RT__Case_Exp__State_initTrial__LC.vi"("input_L_OnOff"=w961, "input_L_Block"=w936, "input_L_Count"=w962, "input_L_Prob"=w963, "input_L_Tdelay"=w964, "input_L_delayOpt"=w965, "input_T_state"=w960, "input_iSpout"=w936, "input_iTrial_relative"=w959, "input_L_T"=w937) -> ("output_LC_Event"=w952:bool, "output_LC_Laser"=w954:bool, "output_L_Tstart"=w953:u16, "output_L_Tend"=w951:u16)  [unwired: 6 in]
            }
          }
          n394 = case shown="1" w481 {
            tunnel: w493 -> [_ w795 w817 w853]
            tunnel: w480 -> [_ w774 w796 w818]
            tunnel: w495 -> [_ w789 w811 w842]
            tunnel: w479 -> [_ w788 w810 w841]
            tunnel: [w772 w787 w799 w840] -> w508
            tunnel: [w772 w786 w799 w839] -> w507
            tunnel: [w773 w785 w798 w838] -> w503
            tunnel: [w773 w784 w798 w837] -> w501
            tunnel: [w772 w777 w809 w836] -> w505
            tunnel: [w773 w776 w808 w835] -> w499
            tunnel: [w772 w777 w807 w834] -> w506
            tunnel: [w773 w776 w806 w833] -> w497
            tunnel: w520 -> [_ w783 _ w832]
            tunnel: w519 -> [_ w782 _ w831]
            tunnel: w518 -> [_ w781 _ w830]
            tunnel: w517 -> [_ w780 _ w829]
            tunnel: w516 -> [_ w779 _ w828]
            tunnel: w515 -> [_ w778 _ w827]
            tunnel: w514 -> [_ _ w805 w826]
            tunnel: w513 -> [_ _ w804 w825]
            tunnel: w512 -> [_ _ w803 w824]
            tunnel: w511 -> [_ _ w802 w823]
            tunnel: w510 -> [_ _ w801 w822]
            tunnel: w509 -> [_ _ w800 w821]
            tunnel: w522 -> [_ w775 _ w820]
            tunnel: w521 -> [_ _ w797 w819]
            frame 0, Default {
              w773 = u16 0
              w772 = FALSE
              # "No active lasers"
            }
            frame 1 {
              w776 = u16 0
              w777 = FALSE
              # "laser1 is active"
              n395 = Index Array(array=w795, index #1=w783, index #2=w782, index #3=w781, index #4=w780, index #5=w779, index #6=w778) -> (element #1=w794:u16, element #3=w793:u16, element #4=w792:u16, element #5=w791:u16, element #6=w790:u16)  [unwired: 1 out]
              n396 = call "BRig_RT__Case_Exp__State_initTrial__LC.vi"("input_L_OnOff"=w794, "input_L_Block"=w774, "input_L_Count"=w793, "input_L_Prob"=w792, "input_L_Tdelay"=w791, "input_L_delayOpt"=w790, "input_T_state"=w789, "input_iSpout"=w774, "input_iTrial_relative"=w788, "input_L_T"=w775) -> ("output_LC_Event"=w787:bool, "output_LC_Laser"=w786:bool, "output_L_Tstart"=w785:u16, "output_L_Tend"=w784:u16)  [unwired: 6 in]
            }
            frame 2 {
              w798 = u16 0
              w799 = FALSE
              # "laser2 is active"
              n397 = Index Array(array=w817, index #1=w805, index #2=w804, index #3=w803, index #4=w802, index #5=w801, index #6=w800) -> (element #1=w812:u16, element #3=w813:u16, element #4=w814:u16, element #5=w815:u16, element #6=w816:u16)  [unwired: 1 out]
              n398 = call "BRig_RT__Case_Exp__State_initTrial__LC.vi"("input_L_OnOff"=w812, "input_L_Block"=w796, "input_L_Count"=w813, "input_L_Prob"=w814, "input_L_Tdelay"=w815, "input_L_delayOpt"=w816, "input_T_state"=w811, "input_iSpout"=w796, "input_iTrial_relative"=w810, "input_L_T"=w797) -> ("output_LC_Event"=w807:bool, "output_LC_Laser"=w809:bool, "output_L_Tstart"=w808:u16, "output_L_Tend"=w806:u16)  [unwired: 6 in]
            }
            frame 3 {
              # "laser1 and laser2 are active"
              n399 = Index Array(array=w853, index #1=w832, index #2=w831, index #3=w830, index #4=w829, index #5=w828, index #6=w827, index #7=w826, index #8=w825, index #9=w824, index #10=w823, index #11=w822, index #12=w821) -> (element #1=w852:u16, element #3=w851:u16, element #4=w850:u16, element #5=w849:u16, element #6=w848:u16, element #7=w843:u16, element #9=w844:u16, element #10=w845:u16, element #11=w846:u16, element #12=w847:u16)  [unwired: 2 out]
              n400 = call "BRig_RT__Case_Exp__State_initTrial__LC.vi"("input_L_OnOff"=w852, "input_L_Block"=w818, "input_L_Count"=w851, "input_L_Prob"=w850, "input_L_Tdelay"=w849, "input_L_delayOpt"=w848, "input_T_state"=w842, "input_iSpout"=w818, "input_iTrial_relative"=w841, "input_L_T"=w820) -> ("output_LC_Event"=w840:bool, "output_LC_Laser"=w839:bool, "output_L_Tstart"=w838:u16, "output_L_Tend"=w837:u16)  [unwired: 6 in]
              n401 = call "BRig_RT__Case_Exp__State_initTrial__LC.vi"("input_L_OnOff"=w843, "input_L_Block"=w818, "input_L_Count"=w844, "input_L_Prob"=w845, "input_L_Tdelay"=w846, "input_L_delayOpt"=w847, "input_T_state"=w842, "input_iSpout"=w818, "input_iTrial_relative"=w841, "input_L_T"=w819) -> ("output_LC_Event"=w834:bool, "output_LC_Laser"=w836:bool, "output_L_Tstart"=w835:u16, "output_L_Tend"=w833:u16)  [unwired: 6 in]
            }
          }
          n402 = call "BRig_dataCurrent_L_ENL_T_start_l1.vi"() -> ("output_L_ENL_T_start_l1"=w564:i32)  [unwired: 11 in]
          n403 = call "BRig_dataCurrent_L_ENL_T_end_l1.vi"() -> ("output_L_ENL_T_end_l1"=w562:i32)  [unwired: 11 in]
          n404 = call "BRig_dataCurrent_L_ENL_T_start_l2.vi"() -> ("output_L_T_ENL1_start_l2"=w560:i32)  [unwired: 11 in]
          n405 = call "BRig_dataCurrent_L_ENL_T_end_l2.vi"() -> ("output_L_ENL_T_end_l2"=w558:i32)  [unwired: 11 in]
          n406 = call "BRig_dataCurrent_L_ENL2_T_start_l1.vi"() -> ("output_L_ENL2_T_start_l1"=w504:i32)  [unwired: 11 in]
          n407 = call "BRig_dataCurrent_L_ENL2_T_end_l1.vi"() -> ("output_L_ENL2_T_end_l1"=w502:i32)  [unwired: 11 in]
          n408 = call "BRig_dataCurrent_L_ENL2_T_start_l2.vi"() -> ("output_L_T_ENL2_start_l2"=w500:i32)  [unwired: 11 in]
          n409 = call "BRig_dataCurrent_L_ENL2_T_end_l2.vi"() -> ("output_L_ENL2_T_end_l2"=w498:i32)  [unwired: 11 in]
          n410 = Replace Array Subset(array=w566, new element #1=w563, index #1=w564, new element #2=w561, index #2=w562, new element #3=w559, index #3=w560, new element #4=w557, index #4=w558, new element #5=w503, index #5=w504, new element #6=w501, index #6=w502, new element #7=w499, index #7=w500, new element #8=w497, index #8=w498) -> (w565:u16[])
          n411 = call "BRig_dataTrial_L_ENL_event_I_l1.vi"() -> ("output_L_ENL_event_I_l1"=w579:i32)  [unwired: 11 in]
          n412 = call "BRig_dataTrial_L_ENL_trig_I_l1.vi"() -> ("output_L_ENL_trig_I_l1"=w576:i32)  [unwired: 11 in]
          n413 = call "BRig_dataTrial_L_ENL_event_I_l2.vi"() -> ("output_L_ENL_event_I_l2"=w575:i32)  [unwired: 11 in]
          n414 = call "BRig_dataTrial_L_ENL_trig_I_l2.vi"() -> ("output_L_ENL_trig_I_l2"=w574:i32)  [unwired: 11 in]
          n415 = call "BRig_dataTrial_L_ENL2_event_I_l1.vi"() -> ("output_L_ENL2_event_I_l1"=w531:i32)  [unwired: 11 in]
          n416 = call "BRig_dataTrial_L_ENL2_trig_I_l1.vi"() -> ("output_L_ENL2_trig_I_l1"=w530:i32)  [unwired: 11 in]
          n417 = call "BRig_dataTrial_L_ENL2_event_I_l2.vi"() -> ("output_L_ENL2_event_I_l2"=w529:i32)  [unwired: 11 in]
          n418 = call "BRig_dataTrial_L_ENL2_trig_I_l2.vi"() -> ("output_L_ENL2_trig_I_l2"=w527:i32)  [unwired: 11 in]
          n419 = call "BRig_arrTrig_L_ENL_event_l1.vi"() -> ("output_L_ENL_event_l1"=w587:i32)  [unwired: 11 in]
          n420 = call "BRig_arrTrig_L_ENL_laser_l1.vi"() -> ("output_L_ENL_laserTrig_l1"=w586:i32)  [unwired: 11 in]
          n421 = call "BRig_arrTrig_L_ENL_event_l2.vi"() -> ("output_L_ENL_event_l2"=w585:i32)  [unwired: 11 in]
          n422 = call "BRig_arrTrig_L_ENL_laser_l2.vi"() -> ("output_L_ENL_laserTrig_l2"=w584:i32)  [unwired: 11 in]
          n423 = call "BRig_arrTrig_L_ENL2_event_l1.vi"() -> ("output_L_ENL2_event_l1"=w539:i32)  [unwired: 11 in]
          n424 = call "BRig_arrTrig_L_ENL2_laser_l1.vi"() -> ("output_L_ENL2_laserTrig_l1"=w538:i32)  [unwired: 11 in]
          n425 = call "BRig_arrTrig_L_ENL2_event_l2.vi"() -> ("output_L_ENL2_event_l2"=w537:i32)  [unwired: 11 in]
          n426 = call "BRig_arrTrig_L_ENL2_laser_l2.vi"() -> ("output_L_ENL2_laserTrig_l2"=w536:i32)  [unwired: 11 in]
          n427 = Boolean To (0,1)(Boolean=w578) -> (0, 1=w583:i16)
          n428 = Boolean To (0,1)(Boolean=w572) -> (0, 1=w582:i16)
          n429 = Boolean To (0,1)(Boolean=w570) -> (0, 1=w580:i16)
          n430 = Boolean To (0,1)(Boolean=w568) -> (0, 1=w581:i16)
          n431 = Boolean To (0,1)(Boolean=w508) -> (0, 1=w535:i16)
          n432 = Boolean To (0,1)(Boolean=w507) -> (0, 1=w534:i16)
          n433 = Boolean To (0,1)(Boolean=w506) -> (0, 1=w532:i16)
          n434 = Boolean To (0,1)(Boolean=w505) -> (0, 1=w533:i16)
          n435 = Replace Array Subset(array=w589, new element #1=w578, index #1=w587, new element #2=w572, index #2=w586, new element #3=w570, index #3=w585, new element #4=w568, index #4=w584, new element #5=w508, index #5=w539, new element #6=w507, index #6=w538, new element #7=w506, index #7=w537, new element #8=w505, index #8=w536) -> (w588:bool[])
          n436 = To Unsigned Word Integer(number=w583) -> (unsigned 16bit integer=w577:u16)
          n437 = To Unsigned Word Integer(number=w582) -> (unsigned 16bit integer=w573:u16)
          n438 = To Unsigned Word Integer(number=w580) -> (unsigned 16bit integer=w571:u16)
          n439 = To Unsigned Word Integer(number=w581) -> (unsigned 16bit integer=w569:u16)
          n440 = To Unsigned Word Integer(number=w535) -> (unsigned 16bit integer=w526:u16)
          n441 = To Unsigned Word Integer(number=w534) -> (unsigned 16bit integer=w525:u16)
          n442 = To Unsigned Word Integer(number=w532) -> (unsigned 16bit integer=w524:u16)
          n443 = To Unsigned Word Integer(number=w533) -> (unsigned 16bit integer=w523:u16)
          n444 = Replace Array Subset(array=w494, new element #1=w577, index (row) #1=w528, index (col) #1=w579, new element #2=w573, index (row) #2=w528, index (col) #2=w576, new element #3=w571, index (row) #3=w528, index (col) #3=w575, new element #4=w569, index (row) #4=w528, index (col) #4=w574, new element #5=w526, index (row) #5=w528, index (col) #5=w531, new element #6=w525, index (row) #6=w528, index (col) #6=w530, new element #7=w524, index (row) #7=w528, index (col) #7=w529, new element #8=w523, index (row) #8=w528, index (col) #8=w527) -> (w567:u16[][])
        }
      }
    }
    frame False {
      w993 = 0
      # "Record laser timing"
      # "Calculate laser timing"
      # "Total Time (ENL)"
      # "iTrial\nrelative"
      # "Total Time (Laser 2)"
      # "Total Time (Laser 1)"
      # "Current directionality, L or R?"
      # "Determine case for\ncalculating laser timing"
      # "2) Get relative iTrial"
      # "1) If Trial Start State = PostReward,\nThen check LC_ENL_nReward"
      # "laser2 active (ENL)?"
      # "laser1 active (ENL)?"
      # "1) If Trial Start State = PostReward,\nThen check LC_ENL_nReward\n\n2) Get relative iTrial"
      # "Gather variables"
      # "Last trial's\niReward\n(0 = not reward)"
      # "nTrials, current block"
      # "idx dataTrial"
      # "Total Time (ENL)"
      # "# PostReward Trials"
      # "Current directionality, L or R?"
      # "Total Time (Laser 2)"
      # "Total Time (Laser 1)"
      # "Calculate settings for ENL"
      # "Set laser settings for ENL and ENL2"
      # "iTrial\nrelative"
      # "laser timing case (ENL)"
      # "Trial start state\n0 (unknown)\n1 (first)\n2 (PreReward)\n3 (PostReward)"
      # "laser2 active?"
      # "laser1 active?"
      n445 = call "BRig_dataCurrent_iSpout.vi"() -> ("output_iSpout"=w1045:i32)  [unwired: 11 in]
      n446 = call "BRig_dataCurrent_LaserSwitch_l1.vi"() -> ("output_LaserSwitch_l1"=w1054:i32)  [unwired: 11 in]
      n447 = call "BRig_dataCurrent_LaserSwitch_l2.vi"() -> ("output_LaserSwitch_l2"=w1053:i32)  [unwired: 11 in]
      n448 = call "BRig_dataCurrent_iTrial.vi"() -> ("output_iTrial"=w994:i32)  [unwired: 11 in]
      n449 = call "BRig_dataExp_L_Ttotal_l1.vi"() -> ("output_L_Ttotal_l1"=w998:i32)  [unwired: 11 in]
      n450 = call "BRig_dataExp_L_Ttotal_l2.vi"() -> ("output_L_Ttotal_l2"=w999:i32)  [unwired: 11 in]
      n451 = call "BRig_dataTrial_sTrial_start.vi"() -> ("output_sTrial_start"=w1050:i32)  [unwired: 11 in]
      n452 = call "BRig_dataTrial_iTrial_PostR.vi"() -> ("output_iTrial_PostR"=w995:i32)  [unwired: 11 in]
      n453 = call "BRig_dataTrial_T_ENL.vi"() -> ("output_T_ENL"=w996:i32)  [unwired: 11 in]
      n454 = Index Array(array=w1021, index #1=w1045, index #2=w1054, index #3=w1053, index #4=w994) -> (element #1=w990:u16, element #2=w1052:u16, element #3=w1051:u16, element #4=w979:u16)
      n455 = Index Array(array=w997, index #1=w998, index #2=w999) -> (element #1=w992:u16, element #2=w991:u16)
      n456 = Index Array(array=w986, index (row) #1=w993, index (col) #1=w1050, index (row) #2=w993, index (col) #2=w995, index (row) #3=w993, index (col) #3=w996) -> (element #1=w977:u16, element #2=w978:u16, element #3=w989:u16)
      n457 = call "BRig_dataTrial_iReward.vi"() -> ("output_iReward"=w987:i32)  [unwired: 11 in]
      n458 = Not Equal To 0?(x=w1052) -> (x != 0?=w982:bool)
      n459 = Not Equal To 0?(x=w1051) -> (x != 0?=w983:bool)
      n460 = Index Array(array=w986, index (row)=1 ("disabled index (row)"), index (col)=w987) -> (element=w985:u16)
      n461 = case shown="3" w977 {
        tunnel: w985 -> [_ _ w1063]
        tunnel: w984 -> [_ _ w1064]
        tunnel: w983 -> [_ w1056 w1058]
        tunnel: w982 -> [_ w1057 w1059]
        tunnel: [w1055 w1057 w1062] -> w975
        tunnel: [w1055 w1056 w1061] -> w974
        frame 0 {
          w1055 = FALSE
        }
        frame 1, Default {
        }
        frame 3 {
          n462 = Boolean To (0,1)(Boolean=w1059) -> (0, 1=w1066:i16)
          n463 = Select(t=i16 2, s=w1058, f=i16 0) -> (s? t:f=w1067:i16)
          n464 = Compound Arithmetic op=ADD(w1066, w1067) -> (w1065:i16)
          n465 = case shown="3" w1065 {
            tunnel: w1064 -> [_ w1074 w1085 w1096]
            tunnel: w1063 -> [_ w1073 w1084 w1095]
            tunnel: [w1070 w1072 w1082 w1094] -> w1062
            tunnel: [w1070 w1071 w1083 w1093] -> w1061
            tunnel: FALSE -> [w1070 w1071 w1082 _]
            frame 0, Default {
            }
            frame 1 {
              n466 = call "BRig_dataLC_ENL_PostR_nRew1_l1.vi"() -> ("output_ENL_PostR_nRew1_l1"=w1081:i32)  [unwired: 11 in]
              n467 = call "BRig_dataLC_ENL_PostR_nRew2_l1.vi"() -> ("output_ENL_PostR_nRew2_l1"=w1080:i32)  [unwired: 11 in]
              n468 = Index Array(array=w1074, index #1=w1081, index #2=w1080) -> (element #1=w1076:u16, element #2=w1075:u16)
              n469 = Equal To 0?(x=w1076) -> (x = 0?=w1077:bool)
              n470 = Equal?(x=w1076, y=w1073) -> (x = y?=w1078:bool)
              n471 = Equal?(x=w1075, y=w1073) -> (x = y?=w1079:bool)
              n472 = Compound Arithmetic op=OR(w1077, w1078, w1079) -> (w1072:bool)
            }
            frame 2 {
              n473 = call "BRig_dataLC_ENL_PostR_nRew1_l2.vi"() -> ("output_ENL_PostR_nRew1_l2"=w1092:i32)  [unwired: 11 in]
              n474 = call "BRig_dataLC_ENL_PostR_nRew2_l2.vi"() -> ("output_ENL_PostR_nRew2_l2"=w1091:i32)  [unwired: 11 in]
              n475 = Index Array(array=w1085, index #1=w1092, index #2=w1091) -> (element #1=w1086:u16, element #2=w1087:u16)
              n476 = Equal To 0?(x=w1086) -> (x = 0?=w1089:bool)
              n477 = Equal?(x=w1086, y=w1084) -> (x = y?=w1088:bool)
              n478 = Equal?(x=w1087, y=w1084) -> (x = y?=w1090:bool)
              n479 = Compound Arithmetic op=OR(w1089, w1088, w1090) -> (w1083:bool)
            }
            frame 3 {
              n480 = call "BRig_dataLC_ENL_PostR_nRew1_l1.vi"() -> ("output_ENL_PostR_nRew1_l1"=w1110:i32)  [unwired: 11 in]
              n481 = call "BRig_dataLC_ENL_PostR_nRew2_l1.vi"() -> ("output_ENL_PostR_nRew2_l1"=w1109:i32)  [unwired: 11 in]
              n482 = call "BRig_dataLC_ENL_PostR_nRew1_l2.vi"() -> ("output_ENL_PostR_nRew1_l2"=w1108:i32)  [unwired: 11 in]
              n483 = call "BRig_dataLC_ENL_PostR_nRew2_l2.vi"() -> ("output_ENL_PostR_nRew2_l2"=w1107:i32)  [unwired: 11 in]
              n484 = Index Array(array=w1096, index #1=w1110, index #2=w1109, index #3=w1108, index #4=w1107) -> (element #1=w1100:u16, element #2=w1099:u16, element #3=w1097:u16, element #4=w1098:u16)
              n485 = Equal To 0?(x=w1100) -> (x = 0?=w1101:bool)
              n486 = Equal?(x=w1100, y=w1095) -> (x = y?=w1102:bool)
              n487 = Equal?(x=w1099, y=w1095) -> (x = y?=w1103:bool)
              n488 = Equal To 0?(x=w1097) -> (x = 0?=w1105:bool)
              n489 = Equal?(x=w1097, y=w1095) -> (x = y?=w1104:bool)
              n490 = Equal?(x=w1098, y=w1095) -> (x = y?=w1106:bool)
              n491 = Compound Arithmetic op=OR(w1101, w1102, w1103) -> (w1094:bool)
              n492 = Compound Arithmetic op=OR(w1105, w1104, w1106) -> (w1093:bool)
            }
          }
        }
      }
      n493 = case shown="3" w977 {
        tunnel: [w1122 w1134 w1146] -> w1011
        tunnel: [w1121 w1133 w1135] -> w1010
        tunnel: [w1120 w1132 w1136] -> w1009
        tunnel: [w1119 w1131 w1137] -> w1008
        tunnel: [w1118 w1130 w1138] -> w1007
        tunnel: [w1117 w1129 w1139] -> w1006
        tunnel: [w1116 w1128 w1145] -> w1005
        tunnel: [w1115 w1127 w1144] -> w1004
        tunnel: [w1114 w1126 w1143] -> w1003
        tunnel: [w1113 w1125 w1142] -> w1002
        tunnel: [w1112 w1124 w1141] -> w1001
        tunnel: [w1111 w1123 w1140] -> w1000
        frame 1, Default {
          n494 = call "BRig_dataLC_ENL_First_OnOff_l1.vi"() -> ("output_ENL_First_OnOff"=w1122:i32)  [unwired: 11 in]
          n495 = call "BRig_dataLC_ENL_First_Block_l1.vi"() -> ("output_ENL_First_Block"=w1121:i32)  [unwired: 11 in]
          n496 = call "BRig_dataLC_ENL_First_Count_l1.vi"() -> ("output_ENL_First_Count"=w1120:i32)  [unwired: 11 in]
          n497 = call "BRig_dataLC_ENL_First_Prob_l1.vi"() -> ("output_ENL_First_Prob"=w1119:i32)  [unwired: 11 in]
          n498 = call "BRig_dataLC_ENL_First_Delay_l1.vi"() -> ("output_ENL_First_Delay"=w1118:i32)  [unwired: 11 in]
          n499 = call "BRig_dataLC_ENL_First_DelayOpt_l1.vi"() -> ("output_ENL_First_DelayOpt"=w1117:i32)  [unwired: 11 in]
          n500 = call "BRig_dataLC_ENL_First_OnOff_l2.vi"() -> ("output_ENL_First_OnOff_l2"=w1116:i32)  [unwired: 11 in]
          n501 = call "BRig_dataLC_ENL_First_Block_l2.vi"() -> ("output_ENL_First_Block_l2"=w1115:i32)  [unwired: 11 in]
          n502 = call "BRig_dataLC_ENL_First_Count_l2.vi"() -> ("output_ENL_First_Count_l2"=w1114:i32)  [unwired: 11 in]
          n503 = call "BRig_dataLC_ENL_First_Prob_l2.vi"() -> ("output_ENL_First_Prob_l2"=w1113:i32)  [unwired: 11 in]
          n504 = call "BRig_dataLC_ENL_First_Delay_l2.vi"() -> ("output_ENL_First_Delay_l2"=w1112:i32)  [unwired: 11 in]
          n505 = call "BRig_dataLC_ENL_First_DelayOpt_l2.vi"() -> ("output_ENL_First_DelayOpt_l2"=w1111:i32)  [unwired: 11 in]
        }
        frame 2 {
          n506 = call "BRig_dataLC_ENL_PreR_OnOff_l1.vi"() -> ("output_ENL_PreR_OnOff"=w1134:i32)  [unwired: 11 in]
          n507 = call "BRig_dataLC_ENL_PreR_Block_l1.vi"() -> ("output_ENL_PreR_Block"=w1133:i32)  [unwired: 11 in]
          n508 = call "BRig_dataLC_ENL_PreR_Count_l1.vi"() -> ("output_ENL_PreR_Count"=w1132:i32)  [unwired: 11 in]
          n509 = call "BRig_dataLC_ENL_PreR_Prob_l1.vi"() -> ("output_ENL_PreR_Prob"=w1131:i32)  [unwired: 11 in]
          n510 = call "BRig_dataLC_ENL_PreR_Delay_l1.vi"() -> ("output_ENL_PreR_Delay"=w1130:i32)  [unwired: 11 in]
          n511 = call "BRig_dataLC_ENL_PreR_DelayOpt_l1.vi"() -> ("output_ENL_PreR_DelayOpt"=w1129:i32)  [unwired: 11 in]
          n512 = call "BRig_dataLC_ENL_PreR_OnOff_l2.vi"() -> ("output_ENL_PreR_OnOff_l2"=w1128:i32)  [unwired: 11 in]
          n513 = call "BRig_dataLC_ENL_PreR_Block_l2.vi"() -> ("output_ENL_PreR_Block_l2"=w1127:i32)  [unwired: 11 in]
          n514 = call "BRig_dataLC_ENL_PreR_Count_l2.vi"() -> ("output_ENL_PreR_Count_l2"=w1126:i32)  [unwired: 11 in]
          n515 = call "BRig_dataLC_ENL_PreR_Prob_l2.vi"() -> ("output_ENL_PreR_Prob_l2"=w1125:i32)  [unwired: 11 in]
          n516 = call "BRig_dataLC_ENL_PreR_Delay_l2.vi"() -> ("output_ENL_PreR_Delay_l2"=w1124:i32)  [unwired: 11 in]
          n517 = call "BRig_dataLC_ENL_PreR_DelayOpt_l2.vi"() -> ("output_ENL_PreR_DelayOpt_l2"=w1123:i32)  [unwired: 11 in]
        }
        frame 3 {
          n518 = call "BRig_dataLC_ENL_PostR_OnOff_l1.vi"() -> ("output_ENL_PostR_OnOff"=w1146:i32)  [unwired: 11 in]
          n519 = call "BRig_dataLC_ENL_PostR_Block_l1.vi"() -> ("output_ENL_PostR_Block"=w1135:i32)  [unwired: 11 in]
          n520 = call "BRig_dataLC_ENL_PostR_Count_l1.vi"() -> ("output_ENL_PostR_Count"=w1136:i32)  [unwired: 11 in]
          n521 = call "BRig_dataLC_ENL_PostR_Prob_l1.vi"() -> ("output_ENL_PostR_Prob"=w1137:i32)  [unwired: 11 in]
          n522 = call "BRig_dataLC_ENL_PostR_Delay_l1.vi"() -> ("output_ENL_PostR_Delay"=w1138:i32)  [unwired: 11 in]
          n523 = call "BRig_dataLC_ENL_PostR_DelayOpt_l1.vi"() -> ("output_ENL_PostR_DelayOpt"=w1139:i32)  [unwired: 11 in]
          n524 = call "BRig_dataLC_ENL_PostR_OnOff_l2.vi"() -> ("output_ENL_PostR_OnOff_l2"=w1145:i32)  [unwired: 11 in]
          n525 = call "BRig_dataLC_ENL_PostR_Block_l2.vi"() -> ("output_ENL_PostR_Block_l2"=w1144:i32)  [unwired: 11 in]
          n526 = call "BRig_dataLC_ENL_PostR_Count_l2.vi"() -> ("output_ENL_PostR_Count_l2"=w1143:i32)  [unwired: 11 in]
          n527 = call "BRig_dataLC_ENL_PostR_Prob_l2.vi"() -> ("output_ENL_PostR_Prob_l2"=w1142:i32)  [unwired: 11 in]
          n528 = call "BRig_dataLC_ENL_PostR_Delay_l2.vi"() -> ("output_ENL_PostR_Delay_l2"=w1141:i32)  [unwired: 11 in]
          n529 = call "BRig_dataLC_ENL_PostR_DelayOpt_l2.vi"() -> ("output_ENL_PostR_DelayOpt_l2"=w1140:i32)  [unwired: 11 in]
        }
      }
      n530 = Less?(x=w977, y=u16 3) -> (x < y?=w980:bool)
      n531 = Select(t=w979, s=w980, f=w978) -> (s? t:f=w976:u16)
      n532 = Boolean To (0,1)(Boolean=w975) -> (0, 1=w1047:i16)
      n533 = Select(t=i16 2, s=w974, f=i16 0) -> (s? t:f=w1048:i16)
      n534 = Add(x=w1047, y=w1048) -> (x+y=w973:i16)
      n535 = case shown="2" w973 {
        tunnel: w984 -> [_ w1177 w1200 w1238]
        tunnel: w990 -> [_ w1169 w1192 w1224]
        tunnel: w989 -> [_ w1170 w1193 w1225]
        tunnel: w976 -> [_ w1168 w1191 w1223]
        tunnel: [w1147 w1167 w1180 w1222] -> w1033
        tunnel: [w1147 w1166 w1180 w1221] -> w1027
        tunnel: [w1148 w1165 w1179 w1220] -> w1018
        tunnel: [w1148 w1164 w1179 w1219] -> w1016
        tunnel: [w1147 w1151 w1190 w1218] -> w1023
        tunnel: [w1148 w1150 w1189 w1217] -> w1014
        tunnel: [w1147 w1151 w1188 w1216] -> w1025
        tunnel: [w1148 w1150 w1187 w1215] -> w1012
        tunnel: w1011 -> [_ w1163 _ w1214]
        tunnel: w1010 -> [_ w1162 _ w1213]
        tunnel: w1009 -> [_ w1161 _ w1212]
        tunnel: w1008 -> [_ w1160 _ w1211]
        tunnel: w1007 -> [_ w1159 _ w1210]
        tunnel: w1006 -> [_ w1158 _ w1209]
        tunnel: w1005 -> [_ w1157 w1186 w1208]
        tunnel: w1004 -> [_ w1156 w1185 w1207]
        tunnel: w1003 -> [_ w1155 w1184 w1206]
        tunnel: w1002 -> [_ w1154 w1183 w1205]
        tunnel: w1001 -> [_ w1153 w1182 w1204]
        tunnel: w1000 -> [_ w1152 w1181 w1203]
        tunnel: w992 -> [_ w1149 _ w1202]
        tunnel: w991 -> [_ _ w1178 w1201]
        frame 0, Default {
          w1148 = u16 0
          w1147 = FALSE
          # "No active lasers"
        }
        frame 1 {
          w1150 = u16 0
          w1151 = FALSE
          # "laser1 is active"
          n536 = Index Array(array=w1177, index #1=w1163, index #2=w1162, index #3=w1161, index #4=w1160, index #5=w1159, index #6=w1158, index #7=w1157, index #8=w1156, index #9=w1155, index #10=w1154, index #11=w1153, index #12=w1152) -> (element #1=w1176:u16, element #2=w1175:u16, element #3=w1174:u16, element #4=w1173:u16, element #5=w1172:u16, element #6=w1171:u16)  [unwired: 6 out]
          n537 = call "BRig_RT__Case_Exp__State_initTrial__LC.vi"("input_L_OnOff"=w1176, "input_L_Block"=w1175, "input_L_Count"=w1174, "input_L_Prob"=w1173, "input_L_Tdelay"=w1172, "input_L_delayOpt"=w1171, "input_T_state"=w1170, "input_iSpout"=w1169, "input_iTrial_relative"=w1168, "input_L_T"=w1149) -> ("output_LC_Event"=w1167:bool, "output_LC_Laser"=w1166:bool, "output_L_Tstart"=w1165:u16, "output_L_Tend"=w1164:u16)  [unwired: 6 in]
        }
        frame 2 {
          w1179 = u16 0
          w1180 = FALSE
          # "laser2 is active"
          n538 = Index Array(array=w1200, index #1=w1186, index #2=w1185, index #3=w1184, index #4=w1183, index #5=w1182, index #6=w1181) -> (element #1=w1194:u16, element #2=w1195:u16, element #3=w1196:u16, element #4=w1197:u16, element #5=w1198:u16, element #6=w1199:u16)
          n539 = call "BRig_RT__Case_Exp__State_initTrial__LC.vi"("input_L_OnOff"=w1194, "input_L_Block"=w1195, "input_L_Count"=w1196, "input_L_Prob"=w1197, "input_L_Tdelay"=w1198, "input_L_delayOpt"=w1199, "input_T_state"=w1193, "input_iSpout"=w1192, "input_iTrial_relative"=w1191, "input_L_T"=w1178) -> ("output_LC_Event"=w1188:bool, "output_LC_Laser"=w1190:bool, "output_L_Tstart"=w1189:u16, "output_L_Tend"=w1187:u16)  [unwired: 6 in]
        }
        frame 3 {
          # "laser1 and laser2 are active"
          n540 = Index Array(array=w1238, index #1=w1214, index #2=w1213, index #3=w1212, index #4=w1211, index #5=w1210, index #6=w1209, index #7=w1208, index #8=w1207, index #9=w1206, index #10=w1205, index #11=w1204, index #12=w1203) -> (element #1=w1237:u16, element #2=w1236:u16, element #3=w1235:u16, element #4=w1234:u16, element #5=w1233:u16, element #6=w1232:u16, element #7=w1226:u16, element #8=w1227:u16, element #9=w1228:u16, element #10=w1229:u16, element #11=w1230:u16, element #12=w1231:u16)
          n541 = call "BRig_RT__Case_Exp__State_initTrial__LC.vi"("input_L_OnOff"=w1237, "input_L_Block"=w1236, "input_L_Count"=w1235, "input_L_Prob"=w1234, "input_L_Tdelay"=w1233, "input_L_delayOpt"=w1232, "input_T_state"=w1225, "input_iSpout"=w1224, "input_iTrial_relative"=w1223, "input_L_T"=w1202) -> ("output_LC_Event"=w1222:bool, "output_LC_Laser"=w1221:bool, "output_L_Tstart"=w1220:u16, "output_L_Tend"=w1219:u16)  [unwired: 6 in]
          n542 = call "BRig_RT__Case_Exp__State_initTrial__LC.vi"("input_L_OnOff"=w1226, "input_L_Block"=w1227, "input_L_Count"=w1228, "input_L_Prob"=w1229, "input_L_Tdelay"=w1230, "input_L_delayOpt"=w1231, "input_T_state"=w1225, "input_iSpout"=w1224, "input_iTrial_relative"=w1223, "input_L_T"=w1201) -> ("output_LC_Event"=w1216:bool, "output_LC_Laser"=w1218:bool, "output_L_Tstart"=w1217:u16, "output_L_Tend"=w1215:u16)  [unwired: 6 in]
        }
      }
      n543 = call "BRig_dataCurrent_L_ENL_T_start_l1.vi"() -> ("output_L_ENL_T_start_l1"=w1019:i32)  [unwired: 11 in]
      n544 = call "BRig_dataCurrent_L_ENL_T_end_l1.vi"() -> ("output_L_ENL_T_end_l1"=w1017:i32)  [unwired: 11 in]
      n545 = call "BRig_dataCurrent_L_ENL_T_start_l2.vi"() -> ("output_L_T_ENL1_start_l2"=w1015:i32)  [unwired: 11 in]
      n546 = call "BRig_dataCurrent_L_ENL_T_end_l2.vi"() -> ("output_L_ENL_T_end_l2"=w1013:i32)  [unwired: 11 in]
      n547 = Replace Array Subset(array=w1021, new element #1=w1018, index #1=w1019, new element #2=w1016, index #2=w1017, new element #3=w1014, index #3=w1015, new element #4=w1012, index #4=w1013) -> (w1020:u16[])
      n548 = call "BRig_dataTrial_L_ENL_event_I_l1.vi"() -> ("output_L_ENL_event_I_l1"=w1034:i32)  [unwired: 11 in]
      n549 = call "BRig_dataTrial_L_ENL_trig_I_l1.vi"() -> ("output_L_ENL_trig_I_l1"=w1031:i32)  [unwired: 11 in]
      n550 = call "BRig_dataTrial_L_ENL_event_I_l2.vi"() -> ("output_L_ENL_event_I_l2"=w1030:i32)  [unwired: 11 in]
      n551 = call "BRig_dataTrial_L_ENL_trig_I_l2.vi"() -> ("output_L_ENL_trig_I_l2"=w1029:i32)  [unwired: 11 in]
      n552 = call "BRig_arrTrig_L_ENL_event_l1.vi"() -> ("output_L_ENL_event_l1"=w1042:i32)  [unwired: 11 in]
      n553 = call "BRig_arrTrig_L_ENL_laser_l1.vi"() -> ("output_L_ENL_laserTrig_l1"=w1041:i32)  [unwired: 11 in]
      n554 = call "BRig_arrTrig_L_ENL_event_l2.vi"() -> ("output_L_ENL_event_l2"=w1040:i32)  [unwired: 11 in]
      n555 = call "BRig_arrTrig_L_ENL_laser_l2.vi"() -> ("output_L_ENL_laserTrig_l2"=w1039:i32)  [unwired: 11 in]
      n556 = Boolean To (0,1)(Boolean=w1033) -> (0, 1=w1038:i16)
      n557 = Boolean To (0,1)(Boolean=w1027) -> (0, 1=w1037:i16)
      n558 = Boolean To (0,1)(Boolean=w1025) -> (0, 1=w1035:i16)
      n559 = Boolean To (0,1)(Boolean=w1023) -> (0, 1=w1036:i16)
      n560 = Replace Array Subset(array=w1044, new element #1=w1033, index #1=w1042, new element #2=w1027, index #2=w1041, new element #3=w1025, index #3=w1040, new element #4=w1023, index #4=w1039) -> (w1043:bool[])
      n561 = To Unsigned Word Integer(number=w1038) -> (unsigned 16bit integer=w1032:u16)
      n562 = To Unsigned Word Integer(number=w1037) -> (unsigned 16bit integer=w1028:u16)
      n563 = To Unsigned Word Integer(number=w1035) -> (unsigned 16bit integer=w1026:u16)
      n564 = To Unsigned Word Integer(number=w1036) -> (unsigned 16bit integer=w1024:u16)
      n565 = Replace Array Subset(array=w986, new element #1=w1032, index (row) #1=w993, index (col) #1=w1034, new element #2=w1028, index (row) #2=w993, index (col) #2=w1031, new element #3=w1026, index (row) #3=w993, index (col) #3=w1030, new element #4=w1024, index (row) #4=w993, index (col) #4=w1029) -> (w1022:u16[][])
    }
  }
  "output_dataCurrent" <- w11
  "output_arrTrig" <- w14
  "output_dataTrial" <- w13
